vi "AlliGator Phasor Graph Actions.vi"(0 "AlliGator Q Elements in":T4[](array[typedef]), 1 "VI in":refnum<vi>, 2 "Script in":bool, 5 "Data Value Reference in":refnum<data-value>, 7 "AlliGator Q Event in":T5=enum."GUI:Idle", 9 "Data":variant, 11 "error in (no error)":errorcluster, 12 "AlliGator Ctrl Refnums":T6) -> (3 "Script out":bool, 4 "AlliGator Q Elements out":T4[](array[typedef]), 6 "Data Value Reference out":refnum<data-value>, 10 "[Notebook Message]":T1[](array[typedef]) {"Message Style"."Text Alignment" items=["Left", "Right", "Center"]}, 15 "error out":errorcluster)   [LabVIEW 2021, in "AlliGator Action Engine.lvlib"]
doc: "Processes AlliGator phasor graph-related actions."
uses:
  AlliGator Action Engine.lvlib
  AlliGator Internal Variables v2.ctl
  <vilib>/vision/Image Controls.llb/IMAQ Image.ctl
  AlliGator Gate Image Set.ctl
  AlliGator FLI Dataset Type.ctl
  AlliGator Data Series Type.ctl
  AlliGator Dataset Channel.ctl
  AlliGator Gate Arithmetic.ctl
  AlliGator Displayed Image.ctl
  Image/Named ROI Description.ctl
  AlliGator Decay Metadata v3.ctl
  AlliGator Decay Background Subtraction Info.ctl
  AlliGator Baseline Subtraction Method.ctl
  Graphs/XY Graph/XY Graph Plot Shift Parameters.ctl
  Graphs/XY Graph/XY Graph Plot Shift Method.ctl
  AlliGator Decay Extrapolation Parameters.ctl
  Phasor/Calibration Phasor (m, phi).ctl
  Phasor/Phasor Reference Series.ctl
  Phasor/Phasor Calibration Map v2.ctl
  Phasor/Phasor (g, s).ctl
  AlliGator Raw Phasor Plot Data v4.ctl
  Phasor/Phasor Standard Deviation Options.ctl
  AlliGator Phasor Multi-Harmonic Data.ctl
  Phasor/Phasor Harmonic Data.ctl
  AlliGator Decay Fit Options & Parameters v2.ctl
  Fits/IRF(X)PSED/Decay Fit Options v2.ctl
  Fits/Decay Convolution/Decay Model.ctl
  Fits/Residual Type.ctl
  Fits/IRF(X)PSED/Fit Weights Type.ctl
  Fits/Non-linear Fitting Method v2.ctl
  Fits/Fit Calculation Method.ctl
  Fits/Non-linear Fitting Algorithm.ctl
  AlliGator Decay Fit Parameter Constraints 2.ctl
  Fits/IRF(X)PSED/Decay Fit Parameters In List.ctl
  Fits/IRF(X)PSED/MLE Baseline Offset Type.ctl
  AlliGator Decay Preprocessing Parameters.ctl
  Fits/IRF(X)PSED/Decay Fit Parameters & Derived Quantities List.ctl
  AlliGator Q Event.ctl
  AlliGator Ctrl Refnums.ctl
  AlliGator Other Ctrl Refnums.ctl
  AlliGator State Indicator.ctl
  AlliGator Phasor Plot Ctrl Refnums.ctl
  AlliGator Phasor Graph Ctrl Refnums.ctl
  Phasor/Phasor Calibration Type.ctl
  AlliGator Dataset Ctrl Refnums.ctl
  AlliGator Registered Events Ctrl Refnums.ctl
  AlliGator Image Histogram Control Refnums.ctl
  Histograms/Linear Histogram Options.ctl
  Histograms/Histogram Bin Option.ctl
  Histograms/Histogram Bin Position.ctl
  AlliGator Decay Fit Map Control Refnums.ctl
  AlliGator Q Element.ctl
  Notebook/Notebook Message Object.ctl
  Rich Text Box/Text Formatting.ctl
  Rich Text Box/Text Colors.ctl
  Graphs/XY Graph/XY Graph Mouse Click Event Data.ctl
  Graphs/XY Graph/XY Graph Refnum.ctl
  <vilib>/Utility/miscctls.llb/LVPoint32TypeDef.ctl
  Graphs/XY Graph/XY Graph Selected Plot Info.ctl
  AlliGator Raw Phasor Plot Array Action.ctl
  Alligator Elements Order in Action Stack.ctl
  Graphs/XY Graph/New Plot Information.ctl
  Graphs/Plot Scales.ctl
  Graphs/LabVIEW Plot Interpolation.ctl
  Graphs/Plot Point Style.ctl
  AlliGator Variables List.ctl
  AlliGator Phasor Plot Scatter Plot Parameters.ctl
  AlliGator Phasor Graph Parameter List.ctl
  AlliGator Phasor Reference Data.ctl
  Phasor/Phasor (m, phi).ctl
  c0cd7910-0c77-40da-ae9a-85fce9394af2.vi
  da8c548c-3fe3-4ac5-84e2-54aef6c91d4f.vi
  Graphs/Get Plot at Mouse Click (XY Graph)/Get Plot at Mouse Click [AAC].vi
  AlliGator Add Single Action to Stack.vi
  AlliGator Add Action Array to Stack.vi
  Variant/Variant to Data/Variant to Boolean.vi
  Variant/Variant to Data/Variant to Path.vi
  Variant/Variant to Data/Variant to [Path].vi
  Arrays/Signed Array Index.vi
  Variant/Variant to Data/Variant to I32.vi
  <vilib>/Utility/error.llb/Error Cluster From Error Code.vi
  Variant/Variant to Data/Variant to U32.vi
  <userlib>/_OpenG.lib/array/array.llb/Filter 1D Array with Scalar (I32)__ogtk.vi
  <vilib>/ErrorRing/Error Ring.xnode
  GUI/GUI.lvlib
  AlliGator Scripts.lvlib
  Graphs/Graphs.lvlib
  Variant/Variant to Data/Variant to Data.lvlib
  AlliGator Phasor Graph.lvlib
  AlliGator Internal Variables.lvlib
  Graphs/XY Graph/XY Graph Add-Ons.lvlib
  Phasor/Phasor.lvlib
  AlliGator Phasor Ratio.lvlib
  Strings/Strings.lvlib
  <userlib>/_OpenG.lib/array/array.llb/openg_array.lvlib
  AlliGator Source Image.lvlib
  AlliGator Files.lvlib
  AlliGator Graphs.lvlib
  AlliGator Settings.lvlib
  Rich Text Box/Rich Text Box.lvlib
  Sound/Sound.lvlib
  Error/Error.lvlib
  AlliGator Globals, Variables & Constants.lvlib
  Image/Image.lvlib
  AlliGator Decay Preprocessing.lvlib
  AlliGator Phasor Plot.lvlib
  Fits/Fits.lvlib
  AlliGator Decay Fit.lvlib
  AlliGator Decay Fit Parameter Map.lvlib
  AlliGator GUI.lvlib
  AlliGator Dual-Channel Datasets.lvlib
  Histograms/Histogram Window.lvlib
  Notebook/Notebook.lvlib
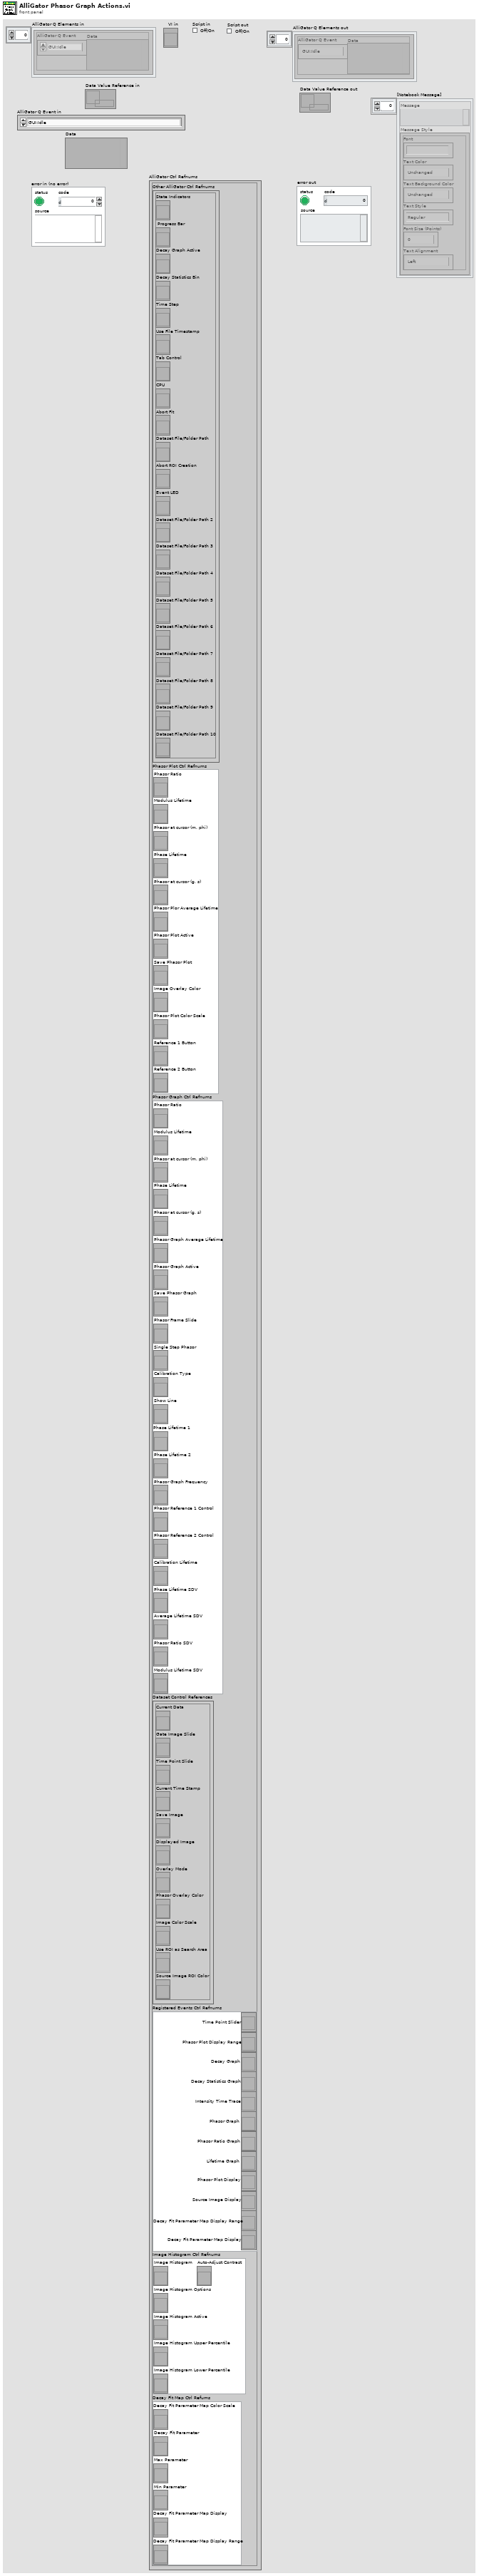
[diagram p1: front panel]
types:
  T1 = typedef "Notebook.lvlib/Notebook Message Object.ctl" = cluster{"Message":string, "Message Style":T2}
  T2 = typedef "Rich Text Box.lvlib/Text Formatting.ctl" = cluster{"Font":string, "Text Color":T3, "Text Background Color":T3, "Text Style":enum16{"Regular", "Bold", "Italic", "Underline", "Strikeout"}, "Font Size (Points)":dbl, "Text Alignment":i32}
  T3 = typedef "Rich Text Box.lvlib/Text Colors.ctl" = enum16{"Unchanged", "Black", "Blue", "Brown", "Gray", "Green", "Orange", "Pink", "Red", "White"}
  T4 = typedef "AlliGator Action Engine.lvlib/AlliGator Q Element.ctl" = cluster{"AlliGator Q Event":T5, "Data":variant}
  T5 = typedef "AlliGator Action Engine.lvlib/AlliGator Q Event.ctl" = enum16{"---- Files ----", "Files:Set Batch Export Files To Save", "Files:Set Dataset Loading & Pre-processing Options", "Files:Check #Frames in Dataset", "Files:Increment Frame Index", "Files:Open Mask Image", "Files:Open White Light Image", "Files:Open Single Dataset", "Files:New Folder of Folders Selected", "Files:Load File (all Types)_Scriptable", "Files:Move Flattened Series to Folders Series", "Files:Select Folder", "Files:Load FLI Dataset", "Files:Load Swiss SPAD 1 Dataset", "Files:Load Swiss SPAD 2 Dataset", "Files:Load .sdt FLI Dataset", "Files:Load .ptu FLI Dataset", "Files:Load .bin FLI Dataset", "Files:Load Single Gate Image Folder", "Files:Load I/m/phi Dataset (deprecated)", "Files:Load Single Image", "Files:Subtract Background File", "Files:Export FLI Dataset", "Files:Load HDF5 FLI Dataset", "Files:Set Destination File Path", "Files:Save Mask Image", "Files:Batch Conversion", "Files:New Folder Selected", "Files:Close FLI Dataset", "Files:Close FLI Dataset Series", "Files:Close White Light Image", "Files:Close Mask Image", "---- FLI Dataset ----", "FLI Dataset:Channel Arithmetic", "FLI Dataset:Export Average Lifetime Map as ASCII", "FLI Dataset:Export User-Defined Quantity Map as ASCII", "FLI Dataset:Python Function FLI Dataset Event", "FLI Dataset:ROI Analysis", "FLI Dataset:Tilted Logistic Square Gated IRF Characteristics Map", "FLI Dataset:Logistic Square Gated IRF Characteristics Map", "FLI Dataset:Square Gated IRF Characteristics Map", "FLI Dataset:Multi-ROI Single-Pixel Phasor Analysis", "FLI Dataset:Multi-ROI Single-Pixel NLSF Analysis", "FLI Dataset:All ROIs IRF Extraction", "FLI Dataset:All ROIs Decay Fit Non-Interactive (Fast + Individual IRF)", "FLI Dataset:All ROIs Phasor Analysis", "FLI Dataset:All ROIs Decay Fit", "FLI Dataset:Fluorescence Decay Statistics", "FLI Dataset:Update Decay Statistics Graph", "FLI Dataset:Get Decay from ROI", "FLI Dataset:All ROIs Average Lifetimes", "---- FLI Dataset Series ----", "FLI Dataset Series:Sum All Datasets in Series", "FLI Dataset Series:Add Dataset to Accumulated Dataset", "FLI Dataset Series:Display Accumulated Dataset", "FLI Dataset Series:Clear Dataset Series Sum", "FLI Dataset Series:Time-Series Analysis (NLSF)", "FLI Dataset Series:Time-Series Analysis (Phasor)", "---- Image ----", "Image:Update Image Profile Plots", "Image:Image Histogram Cursor Move", "Image:Image Histogram", "Image:Image Contrast", "Image:Set Image Histogram Cursor Move Flag", "Image:Clear Image Overlay", "Image:Use ROI as Search Area", "Image:Set ROI Diameter", "Image:Save Image Data as TIFF", "Image:Save Displayed Image with Overlay", "Image:Save Image Overlay Only", "Image:Save Image as Hot Pixel Mask", "Image:Change Source Image Color Palette", "Image:Copy Image to Clipboard", "Image:Source Image ROI Selection", "Image:Delete All ROIs", "Image:Delete All Unselected ROIs", "Image:Delete ROI", "Image:Merge All ROIs", "Image:Store ROI", "Image:Source Image ROI Storage", "Image:Export ROI Description to Notebook", "Image:Save ROI", "Image:Load ROI", "Image:Paste ROI Definition", "Image:Clear ROI", "Image:Identify ROIs in Mask Image", "Image:Create Complementary ROI", "Image:Create Contour ROI", "Image:Create ROI(s) from Pixels with Peak above Min_Scriptable", "Image:Create ROI(s) from Pixels with Intensity above Min_Scriptable", "Image:Compute ROI Statistics", "Image:Delete ROI(s) based on ROI Characteristics", "Image:Create ROI Grid", "Image:ROI to Individual Pixel ROIs", "Image:Python Function Source Image Event", "Image:Show Phasor Calibration Map ROI Centers", "Image:Convert ROI to Mask Image", "Image:Mouse Move", "Image:Mouse Up", "Image:Set Source Image Mouse Move Flag", "Image:Add Scale Bar Overlay", "Image:Delete Existing ROIs Option", "---- Decay ----", "Decay:Clear IRF/Reference Plot", "Decay:Clear Local IRFs", "Decay:Add Decay to Graph", "Decay:Smoothen Plot", "Decay:Smoothen Plot Tail", "Decay:Average Selected Plots", "Decay:Extract IRF", "Decay:Optimal IRF Extraction", "Decay:Threshold IRF", "Decay:Fit to Model IRF", "Decay:Fit IRF to Square Gate", "Decay:Fit IRF to Logistic Square Gate", "Decay:Fit IRF to Tilted Logistic Square Gate", "Decay:Create Bounding Cursors Set", "Decay:Export Bounding Cursors Definition to Notebook", "Decay:Denoise Plot", "Decay:Compute Cumulative Function", "Decay:Use as Reference Decay", "Decay:Show Reference Decay/IRF", "Decay:Extrapolate Decay", "Decay:Create Head & Tail Bounding Cursors", "Decay:Store Cursor-defined Head & Tail Fractions", "Decay:Rebin Plot", "Decay:1-Normalize Decay", "Decay:[0-1]-Normalize Plot", "Decay:Straighten Decay", "Decay:Shift Decay", "Decay:Fold Decay", "Decay:Fit Decay", "Decay:Global Fit of Selected Decays", "Decay:Post Global Fit Script", "Decay:Add Global Fit Parameters to Graph", "Decay:Add Decay Parameter(s) to Plot (Graph)", "Decay:Export Decay to Phasor Graph", "Decay:Plot Decay Shifts", "Decay:Compute Average Lifetime", "Decay:Plot Convolution", "Decay:Graph Tip Strip Update", "---- Decay Statistics ----", "Decay Statistics:Tip Strip Update", "---- Intensity Time Trace ----", "Intensity Time Trace:Use File Timestamp", "Intensity Time Trace:Load Intensity Corrections File", "Intensity Time Trace:Clear Intensity Corrections File", "Intensity Time Trace:Tip Strip Update", "---- Phasor Plot ----", "Phasor Plot:Build Phasor Plot", "Phasor Plot:Change Phasor Plot Color Palette", "Phasor Plot:Adjust Phasor Plot Display Range", "Phasor Plot:Highlight Image ROI in Phasor Plot", "Phasor Plot:Save Phasor Plot Image with Overlay", "Phasor Plot:Export Complex Phasor Map", "Phasor Plot:Export Phasor Ratio Map", "Phasor Plot:Export Average Lifetime Map", "Phasor Plot:Compute Phase Lifetime Histogram", "Phasor Plot:Compute Phasor Ratio Histogram", "Phasor Plot:Compute Phase Lifetime vs Intensity Scatter Plot", "Phasor Plot:Weber 2-Component Decomposition", "Phasor Plot:Update Phasor Color Map Vertices", "Phasor Plot:Clear Phasor Overlay", "Phasor Plot:Use Segment Extremities as References", "Phasor Plot:Use UC/Segment Intersections as References", "Phasor Plot:Use UC/Principal Axis Intersections as References", "Phasor Plot:Use UC/Linear Fit Intersections as References", "Phasor Plot:Update Phasor Plot Reference", "Phasor Plot:Show Local Phasor Info in Phasor Plot", "Phasor Plot:Update Phasor Plot State", "Phasor Plot:Phasor Plot ROI Storage", "Phasor Plot:Phasor Plot ROI Selection", "Phasor Plot:Python Function Phasor Plot Event", "Phasor Plot:Overlay Phasor ROI, Ratio or Map in Source Image", "Phasor Plot:Compute Decay of Selected Phasors", "Phasor Plot:Phasor at Image Pixel", "Phasor Plot:Mouse Move", "Phasor Plot:Mouse Up", "Phasor Plot:Display Range Mouse Move", "Phasor Plot:Set Mouse Move Flag", "---- Phasor Graph ----", "Phasor Graph:Calibrated Phasor Map Series", "Phasor Graph:Whole Image Phasor Scatter Plot (Todo)", "Phasor Graph:Get Phasor Value", "Phasor Graph:Create New Phasor Plot Dialog", "Phasor Graph:Update Last Phasor Value", "Phasor Graph:Update Phasor (m, phi)", "Phasor Graph:Remove Single Phasor from Plot", "Phasor Graph:Add Single Phasor to Plot", "Phasor Graph:Remove Phasor Plot", "Phasor Graph:Remove Selected Phasor Plots", "Phasor Graph:Clear Phasor Data", "Phasor Graph:Clear Phasor Graph", "Phasor Graph:Cursor Move", "Phasor Graph:Draw Cursor Connecting Line", "Phasor Graph:Clear Cursor Connecting Line", "Phasor Graph:Find UC Intersection", "Phasor Graph:Use UC/Cursor-Defined Line Intersections", "Phasor Graph:Use Selected Plots Fitted Line/UC Intersections", "Phasor Graph:Use Selected Plots Principal Axis/UC Intersections", "Phasor Graph:Show Single Phasor", "Phasor Graph:Save Single Phasor Plot", "Phasor Graph:Save All Phasor Plots", "Phasor Graph:Load Phasor Plot(s)", "Phasor Graph:Phasor Multiplication", "Phasor Graph:Compute Average Phasor", "Phasor Graph:Compute Multiple Average Phasors (Selected Plots)", "Phasor Graph:Export Single Phasor Plot Phase Lifetimes", "Phasor Graph:Phase Lifetime Trajectory", "Phasor Graph:Phase Lifetime vs Intensity Scatter Plot (deprecated)", "Phasor Graph:Parameter 2 vs Parameter 1 Scatter Plot", "Phasor Graph:Use Cursor n Location", "Phasor Graph:Set Reference n to Current Phase Lifetime Value", "Phasor Graph:Set Reference n to Lifetime Value", "Phasor Graph:Set Cursor n Location", "Phasor Graph:Save Phasor Graph Image", "Phasor Graph:Update SEPL Plot", "Phasor Graph:Export Single Phasor Plot Data", "Phasor Graph:Export Selected Phasor Plots Data", "Phasor Graph:Python Function Phasor Graph Event", "Phasor Graph:Tip Strip Update", "---- Calibration ----", "Calibration:Set Calibration Type", "Calibration:Load/Save Phasor Calibration", "Calibration:Load/Save Phasor Calibration Series", "Calibration:Load/Save Phasor Calibration Map", "Calibration:Use as Calibration", "Calibration:Compute Optimal Calibration from Phasor References", "Calibration:Clear Phasor Calibration", "Calibration:Single Phasor Calibration Information", "Calibration:Use as Calibration Series", "Calibration:Use as Calibration Map", "Calibration:Clear Calibration Series", "Calibration:Phasor Calibration Series Information", "Calibration:Clear Calibration Map", "Calibration:Phasor Calibration Map Information", "Calibration:Apply Phasor Calibration", "Calibration:Update Single Plot Calibration", "Calibration:Update Multiple Plots Calibration", "Calibration:Clear Single Plot Calibration", "Calibration:Clear All Plots Calibrations", "Calibration:Clear Plot(s) Calibration(s)?", "Calibration:Phasor Calibration Maps (# Gates Series)", "---- Phasor Ratio ----", "Phasor Ratio:Clear Reference n", "Phasor Ratio:Toggle Selected Plot(s)  Lock to Reference 1", "Phasor Ratio:Use as Reference n", "Phasor Ratio:Send Reference n to Notebook", "Phasor Ratio:Toggle Selected Plot(s)  Lock to Reference 2", "Phasor Ratio:Compute Phasor Ratio at Mouse Location", "Phasor Ratio:Compute Phasor Plot's Average Phasor Ratio", "Phasor Ratio:Compute Time-Series Phasor Ratios", "Phasor Ratio:Fit Line to Phasor Ratio Plot", "Phasor Ratio:Save References", "Phasor Ratio:Load References", "Phasor Ratio:Update Phasor Reference 1", "Phasor Ratio:Update Phasor Reference 2", "Phasor Ratio:Move Cursor n to Reference n", "Phasor Ratio:Use as Phasor Reference 1 Lifetime", "Phasor Ratio:Use as Phasor Reference 2 Lifetime", "Phasor Ratio:Export Phasor Ratio Map as ASCII", "Phasor Ratio:Tip Strip Update", "---- Lifetime & Other Parameters Graph ----", "Lifetime:Tip Strip Update", "---- Decay Fit Parameter Map ----", "Decay Fit Parameter Map:Export ROI NLSF Data as ASCII", "Decay Fit Parameter Map:Set Decay Fit  Parameter Map Selection", "Decay Fit Parameter Map:Build Decay Fit Parameter Map", "Decay Fit Parameter Map:Change Decay Fit Parameter Map Color Palette", "Decay Fit Parameter Map:Export Decay Fit Parameter Map Data as ASCII", "Decay Fit Parameter Map:Export All Decay Fit Parameter Maps Data as ASCII", "Decay Fit Parameter Map:Send Map Data to Lifetime Graph", "Decay Fit Parameter Map:Save Decay Fit Parameter Map Image", "Decay Fit Parameter Map:Save-Load IRFs & Fit Data", "Decay Fit Parameter Map:Update Local Decay Plots", "Decay Fit Parameter Map:Python Function Decay Fit Parameters Map Event", "Decay Fit Parameter Map:Overlay Decay Fit Parameter Map in Source Image", "Decay Fit Parameter Map:Plot Map Data vs Intensity", "Decay Fit Parameter Map:Mouse Up", "Decay Fit Parameter Map:Display Range Mouse Move", "---- Generic Graph ----", "Generic Graph:Generic XY Graph Event", "Generic Graph:Python Function XY Graph Event", "Generic Graph:New Plot", "Generic Graph:Save Plot", "Generic Graph:XY Plot Histogram", "Generic Graph:Set XY Graph Plot Name", "Generic Graph:Set Last Cursor Style", "Generic Graph:Tip Strip Update", "---- GUI ----", "GUI:Start Script", "GUI:Type of Displayed Image Changed", "GUI:Gate Image Slide Changed", "GUI:Show Busy Icon", "GUI:Show Busy Icon & Abort Button", "GUI:Hide Busy Icon", "GUI:Hide Busy Icon & Abort Button", "GUI:Abort", "GUI:End Script", "GUI:Start Timing", "GUI:End Timing", "GUI:Set State Indicator", "GUI:Send Parameters JSON Strings to Clipboard", "GUI:Set Gate Step", "GUI:Idle", "GUI:Initialization", "GUI:Quit", "GUI:Increment Dataset Index", "GUI:Set Dataset Index to -1", "GUI:Time Series Slider Moved", "GUI:Time Series Slider Changed", "GUI:Toggle Playback or Loop", "GUI:Playback Script", "GUI:Set Phasor Frequency", "GUI:Open Window", "GUI:Start Test Script", "GUI:End Test Script", "DEBUG"}
  T6 = typedef "AlliGator GUI.lvlib/AlliGator Ctrl Refnums.ctl" = cluster{"Other AlliGator Ctrl Refnums":T7, "Phasor Plot Ctrl Refnums":T8, "Phasor Graph Ctrl Refnums":T9, "Dataset Control References":T10, "Registered Events Ctrl Refnums":T11, "Image Histogram Ctrl Refnums":T12, "Decay Fit Map Ctrl Refums":T13}
  T7 = typedef "AlliGator GUI.lvlib/AlliGator Other Ctrl Refnums.ctl" = cluster{"State Indicators":refnum<vi>, " Progress Bar":refnum<vi>, "Decay Graph Active":refnum<vi>, "Decay Statistics Bin":refnum<vi>, "Time Step":refnum<vi>, "Use File Timestamp":refnum<vi>, "Tab Control":refnum<vi>, "CPU":refnum<vi>, "Abort Fit":refnum<vi>, "Dataset File/Folder Path":refnum<vi>, "Abort ROI Creation":refnum<vi>, "Event LED":refnum<vi>, "Dataset File/Folder Path 2":refnum<vi>, "Dataset File/Folder Path 3":refnum<vi>, "Dataset File/Folder Path 4":refnum<vi>, "Dataset File/Folder Path 5":refnum<vi>, "Dataset File/Folder Path 6":refnum<vi>, "Dataset File/Folder Path 7":refnum<vi>, "Dataset File/Folder Path 8":refnum<vi>, "Dataset File/Folder Path 9":refnum<vi>, "Dataset File/Folder Path 10":refnum<vi>}
  T8 = typedef "AlliGator GUI.lvlib/AlliGator Phasor Plot Ctrl Refnums.ctl" = cluster{"Phasor Ratio":refnum<vi>, "Modulus Lifetime":refnum<vi>, "Phasor at cursor (m, phi)":refnum<vi>, "Phase Lifetime":refnum<vi>, "Phasor at cursor (g, s)":refnum<vi>, "Phasor Plor Average Lifetime":refnum<vi>, "Phasor Plot Active":refnum<vi>, "Save Phasor Plot":refnum<vi>, "Image Overlay Color":refnum<vi>, "Phasor Plot Color Scale":refnum<vi>, "Reference 1 Button":refnum<vi>, "Reference 2 Button":refnum<vi>}
  T9 = typedef "AlliGator GUI.lvlib/AlliGator Phasor Graph Ctrl Refnums.ctl" = cluster{"Phasor Ratio":refnum<vi>, "Modulus Lifetime":refnum<vi>, "Phasor at cursor (m, phi)":refnum<vi>, "Phase Lifetime":refnum<vi>, "Phasor at cursor (g, s)":refnum<vi>, "Phasor Graph Average Lifetime":refnum<vi>, "Phasor Graph Active":refnum<vi>, "Save Phasor Graph":refnum<vi>, "Phasor Frame Slide":refnum<vi>, "Single Step Phasor":refnum<vi>, "Calibration Type":refnum<vi>, "Show Line":refnum<vi>, "Phase Lifetime 1":refnum<vi>, "Phase Lifetime 2":refnum<vi>, "Phasor Graph Frequency":refnum<vi>, "Phasor Reference 1 Control":refnum<vi>, "Phasor Reference 2 Control":refnum<vi>, "Calibration Lifetime":refnum<vi>, "Phase Lifetime SDV":refnum<vi>, "Average Lifetime SDV":refnum<vi>, "Phasor Ratio SDV":refnum<vi>, "Modulus Lifetime SDV":refnum<vi>}
  T10 = typedef "AlliGator GUI.lvlib/AlliGator Dataset Ctrl Refnums.ctl" = cluster{"Current Data":refnum<vi>, "Gate Image Slide":refnum<vi>, "Time Point Slide":refnum<vi>, "Current Time Stamp":refnum<vi>, "Save Image":refnum<vi>, "Displayed Image":refnum<vi>, "Overlay Mode":refnum<vi>, "Phasor Overlay Color":refnum<vi>, "Image Color Scale":refnum<vi>, "Use ROI as Search Area":refnum<vi>, "Source Image ROI Color":refnum<vi>}
  T11 = typedef "AlliGator GUI.lvlib/AlliGator Registered Events Ctrl Refnums.ctl" = cluster{"Time Point Slider":refnum<vi>, "Phasor Plot Display Range":refnum<vi>, "Decay Graph":refnum<vi>, "Decay Statistics Graph":refnum<vi>, "Intensity Time Trace":refnum<vi>, "Phasor Graph":refnum<vi>, "Phasor Ratio Graph":refnum<vi>, "Lifetime Graph":refnum<vi>, "Phasor Plot Display":refnum<vi>, "Source Image Display":refnum<vi>, "Decay Fit Parameter Map Display Range":refnum<vi>, "Decay Fit Parameter Map Display":refnum<vi>}
  T12 = typedef "AlliGator GUI.lvlib/AlliGator Image Histogram Control Refnums.ctl" = cluster{"Image Histogram":refnum<vi>, "Image Histogram Options":refnum<vi>, "Image Histogram Active":refnum<vi>, "Image Histogram Upper Percentile":refnum<vi>, "Image Histogram Lower Percentile":refnum<vi>, "Auto-Adjust Contrast":refnum<vi>}
  T13 = typedef "AlliGator Decay Fit Parameter Map.lvlib/AlliGator Decay Fit Map Control Refnums.ctl" = cluster{"Decay Fit Parameter Map Color Scale":refnum<vi>, "Decay Fit Parameter":refnum<vi>, "Max Parameter":refnum<vi>, "Min Parameter":refnum<vi>, "Decay Fit Parameter Map Display":refnum<vi>, "Decay Fit Parameter Map Display Range":refnum<vi>}
  T14 = typedef "XY Graph Add-Ons.lvlib/XY Graph Selected Plot Info.ctl" = cluster{"Multiplot XY Graph":T15, "Mouse Coordinates":T16, "Plot Index":i32}
  T15 = typedef "XY Graph Add-Ons.lvlib/XY Graph Refnum.ctl" = refnum<vi>
  T16 = typedef "LVPoint32TypeDef.ctl" = cluster{"Horizontal":i32, "Vertical":i32}
  T17 = typedef "XY Graph Add-Ons.lvlib/XY Graph Mouse Click Event Data.ctl" = cluster{"Multiplot XY Graph":T15, "Mouse Coordinates":T16}
  T18 = typedef "Phasor.lvlib/Calibration Phasor (m, phi).ctl" = cluster{"m":dbl, "phi":dbl, "Phasor Frequency":dbl[unit], "Reference Lifetime":dbl[unit]}
  T19 = typedef "AlliGator Phasor Graph.lvlib/AlliGator Raw Phasor Plot Array Action.ctl" = enum16{"Clear All", "-", "Add Raw Phasor Plot", "Delete Raw Phasor Plot", "Replace Raw Phasor Plot", "---------------------", "Add Phasor to Plot", "Replace Phasor in Plot", "Remove Phasor in Plot"}
  T20 = typedef "AlliGator Action Engine.lvlib/Alligator Elements Order in Action Stack.ctl" = enum16{"Enqueue 2 AFTER 1", "Enqueue 2 BEFORE 1"}
  T21 = typedef "XY Graph Add-Ons.lvlib/New Plot Information.ctl" = cluster{"Multiplot XY Graph":refnum<vi>, "Plot Name":string, "Plot Scales":T22, "Plot Interpolation":T23, "Point Style":T24, "Plot Color":u32, "Plot Metadata":variant}
  T22 = typedef "XY Graph Add-Ons.lvlib/Plot Scales.ctl" = cluster{"X Scale":u32, "Y Scale":u32}
  T23 = typedef "Graphs.lvlib/LabVIEW Plot Interpolation.ctl" = u8
  T24 = typedef "Graphs.lvlib/Plot Point Style.ctl" = enum16{"not defined", "None", "Empty Circle", "Filled Circle", "Thick Circle", "Dotted Circle", "Empty Square", "Filled Square", "Thick Square", "Dotted Square", "Small Filled Square", "Dot", "Cross", "Tiny Cross", "Large X", "Small x", "Diamond", "Small Empty Square"}
  T25 = typedef "AlliGator Globals, Variables & Constants.lvlib/AlliGator Variables List.ctl" = enum16{"---- GUI ----", "Initialization Status", "State Indicators Refnum", "Original AlliGator Menu Items", "Current Action Loop State", "Script in progress", "Playback", "Loop Playback", "Search ROI Used", "Search ROI", "Decay Graph Max Legend Size", "Intensity Graph Max Legend Size", "Decay Statistics Graph Max Legend Size", "Phasor Graph Max Legend Size", "Phasor Ratio Graph Max Legend Size", "Lifetime Graph Max Legend Size", "---- Files ----", "Export Dataset Frames as Individual Files", "Show Batch Export Help Balloons", "Frames in Dataset", "ptu File Frame Start Indices", "Current Frame in Dataset", "Current Frame Timestamp", "------ Python Plugins ------", "Python Plugins Information", "Python Session", "Valid Python Session?", "---- Source Image ----", "Dataset Loaded", "Dataset Metadata", "Dataset Channel", "Dataset Data Description", "Background Dataset Metadata", "Background Dataset Channel", "Background Dataset Data Description", "Background File Subtraction", "Background File Path", "Background File Pile-up Correction", "Background File Pixel Well Capacity", "Background File Scaling Factor", "Source Image ROIs", "Current Source Image ROI", "Source Image ROI Event Refnum", "X_Source Image Display Range", "X_Source Image Palette Information", "Source Image Palette List", "Source Image Scale", "Current Dataset Load Settings", "Source Image:ROI Overlay Color", "---- Image Profile Window ----", "Image Profile:Overlay ROI in Source Image", "Image Profile Window Event Refnum", "Image Profile:IntensityType", "Image Profile:Intensity Average Type", "Image Profile:Intensity-weighted SDV", "Image Profile:Box Profile Type", "Image Profile Window Open", "Image Profile:Plotted Fit Parameter", "X_Type of Displayed Image", "X_Time Gate Slider", "Dataset Path", "Source Image Overlay to Erase", "Is Displayed Image Accumulated", "White Light Image Modified", "Mask Image Modified", "Macrotime Gate Separation", "------ Phasor Graph -------", "Phasor Graph:Show Line", "---- Phasor Plot ---", "Phasor Plot Parameters Changed", "FLI Dataset Modified since last Phasor Plot Calculation", "Phasor Harmonics Data", "Selected Phasor Harmonics", "Phasor Harmonic Manager Event Refnum", "Phasor Plot ROIs", "Current Phasor Plot ROI", "Phasor Plot ROI Event Refnum", "Phasor Plot Image Reference Points", "Phasor Plot Computed", "Phasor Plot Palette Information", "Phasor Plot Palette List", "Phasor Ratio Palette Information", "Phasor Ratio Palette List", "Phasor Image Scale", "Phasor Plot Image Overlay to Erase", "Phasor Plot Image Elements to Update", "Current Phasor Plot Calculation Parameters", "Current Phasor Calibration Options", "Reset Cumulated Phasor Plot", "Phasor Ratio Reference 1", "Phasor Ratio Lifetime Reference 1", "Phasor Ratio Reference 1 Frequency", "Phasor Ratio Reference 2", "Phasor Ratio Lifetime Reference 2", "Phasor Ratio Reference 2 Frequency", "---- Decay Analysis ----", "Number of Selected Decays to Fit", "LS Fit Results", "LAR Fit Results", "BS Fit Results", "Last Decay Max - Min", "Best Fit Parameters", "Best Fit Parameter Names", "Actual Size X", "Actual Size Y", "Binning X", "Binning Y", "Actual # Gates", "Dataset Number", "Gates to...", "Gates Skipped", "Gates to keep", "Gate Step", "Gate Separation", "Reversed Gates", "Pile-up Correction", "Pixel Well Capacity", "Background Subtracted", "Background Subtraction Method", "Background Definition Range", "Background File (deprecated)", "Number of Dataset Accumulated", "Array of Accumulated Dataset Paths", "Do Averaged Datasets", "Destination File Path", "Process Plot Target", "Use 1/D as Phasor Frequency", "---- Decay Fit Parameter Map -----", "Decay Fit Parameter Map Palette Information", "Decay Fit Parameter Map Palette List", "Local Decay Graph Window Event Refnum", "------- Local Decay Window ---------", "Use normalized IRF for convolution", "----- Miscellaneous ----", "Skippable Dialog Windows Status"}
  T26 = cluster{"Mouse Click Event Data":T17, "Save as...":bool}
  T27 = typedef "AlliGator Phasor Graph.lvlib/AlliGator Phasor Plot Scatter Plot Parameters.ctl" = cluster{"Parameter 2":T28, "Parameter 1":T28}
  T28 = typedef "AlliGator Phasor Graph.lvlib/AlliGator Phasor Graph Parameter List.ctl" = enum16{"Time Stamp", "Index", "Phasor Parameters", "Phasor g", "Phasor s", "Phasor phi", "Phasor m", "Modulus Lifetime", "Phase Lifetime", "ROI Parameters", "ROI Center x", "ROI Center y", "ROI # pixels ", "Decay Parameters", "Intensity", "Background/Gate", "Intensity - Background", "Fitted Lifetime", "Fitted Intensity", "Phasor Ratio Parameters", "Amplitude Phasor Ratio", "Intensity Phasor Ratio", "Amplitude-Averaged Lifetime", "Intensity-Averaged Lifetime", "-", "Phasor Parameters SDV", "Phasor g SDV", "Phasor s SDV", "Phasor phi SDV", "Phasor m SDV", "Phase Lifetime SDV", "Modulus Lifetime SDV", "Phasor Ratio Parameters SDV", "Amplitude Phasor Ratio SDV", "Intensity Phasor Ratio SDV", "Amplitude-Averaged Lifetime SDV", "Intensity-Averaged Lifetime SDV"}
  T29 = typedef "Phasor.lvlib/Phasor (g, s).ctl" = cluster{"g":dbl, "s":dbl}
  T30 = cluster{"Current Phasor (g, s)":T29, "Cursor Id":u32}
  T31 = typedef "AlliGator Phasor Ratio.lvlib/AlliGator Phasor Reference Data.ctl" = cluster{"Data Type":string, "Data":variant}
  T32 = typedef "Phasor.lvlib/Phasor (m, phi).ctl" = cluster{"m":dbl, "phi":dbl}
  T33 = typedef "AlliGator Internal Variables.lvlib/AlliGator Internal Variables v2.ctl" = cluster{"Displayed Image":T34, "White Light Image":T34, "Mask Image":T34, "ROI Mask Image":T34, "Current Dataset Images 1":T35, "Background Dataset Images 1":T35, "Current Dataset Images 2":T35, "Background Dataset Images 2":T35, "Current Dataset Arithmetic Images":T35, "Accumulated Dataset Images 1":T35, "Accumulated Dataset Images 2":T35, "Accumulated Dataset Arithmetic Images":T35, "Phasor Plot Image":T34, "Decay Fit Parameter Map Image":T34, "Single Data Point Path":path, "White Light Image Path":path, "Mask Image Path":path, "Time-Series Folder":path, "[Time-Series Paths]":path[], "Current Dataset":i32, "Single Dataset Type":T36, "Current Folder":string, "AlliGator Data Series Type":T37, "# Datasets":i32, "Dual-Channel Dataset":bool, "Selected Channel Name":string, "Dataset Channel":T38, "Channel Arithmetic":T39, "Dual-Channel Background Dataset":bool, "Background Channel":T38, "Dual-Channel Accumulated Dataset":bool, "Start Time":dbl, "[Time-Series Timestamps]":dbl[], "[Intensity Corrections]":dbl[], "Time Series Script":bool, "Type of Displayed Image":T40, "Gate Image Slide":u16, "# Gates":i32, "ROIs":T41[], "ROI Decay":cluster{"t Array":dbl[], "I Array":dbl[]}, "Valid Decay":bool, "Decay  Metadata":T43, "Reference Decay Plot Name":string, "Reference Decay":cluster{"t Array":dbl[], "I Array":dbl[]}, "Decay Shift Plot":cluster{"Time Stamps":dbl[], "Decay Shifts":dbl[]}, "[Decays Max Values]":sgl[], "[Decays Min Values]":sgl[], "Calibration Phasor":T18, "Calibration Phasor Series":T49, "Phasor Calibration Map":T50, "Calibration Map MD5 Digest":string, "Last Raw Phasor":T29, "Last Calibrated Phasor":T29, "Last Calibrated Phasor SDV":T29, "Phasor Graph:Phasor Plot":cluster{"g Array":dbl[], "s Array":dbl[]}, "Phasor Graph:Phasor SDV Plot":cluster{"g Array":dbl[], "s Array":dbl[]}, "[Phasor Graph:Raw Phasor Plots]":T51[], "Phasor Plot locked to Ref 1":i32, "[Phasor Plot(s) locked to Ref 1]":i32[], "[Phasor Plot(s) locked to Ref 2]":i32[], "[Pixel Phasors]":T29[], "[[Sum Image]]":dbl[][], "[[CSG Phasors]]":csg[][], "[[Valid Pixel?]]":bool[][], "I/m/phi Dataset":cluster{"I/m/phi Dataset?":bool, "Base Frequency":dbl[unit], "Harmonic Orders":u8[]}, "Multi Phasor Plot Data":T53, "Decay Fit Options & Parameters":T55, "Fit Options: Decay Preprocessing Parameters":T66, "Fit Options: Reference Decay":cluster{"t Array":dbl[], "I Array":dbl[]}, "Is Full Image Parameters Map":bool, "Is Single-Pixels Parameters Map":bool, "NLSF Parameters Map X Resolution":i32, "NLSF Parameters Map Y Resolution":i32, "[Single Decay Fit Parameters]":dbl[], "Fit Model":T57, "[[Multiple Decays Fit Parameters]]":dbl[][], "[[Multiple Decays Fit Parameter SDVs]]":dbl[][], "[[IRFs]]":dbl[][], "IRF Array Time Axis":dbl[], "Decay Array Time Axis":dbl[], "[Decay Fit Parameter Names]":T67[], "[[Phasor Ratios]]":dbl[][], "[[Average Lifetimes]]":dbl[][], "Amplitude Weighted Average Lifetime":bool, "[Decay Sum]":dbl[], "[[User-defined Quantities]]":dbl[][], "User-defined Quantity":string}
  T34 = typedef "IMAQ Image.ctl" = refnum<image>
  T35 = typedef "AlliGator Internal Variables.lvlib/AlliGator Gate Image Set.ctl" = cluster{"SGL Image Max":T34, "SGL Image Sum":T34, "SGL Gate Images":T34[], "SGL Image Min":T34}
  T36 = typedef "AlliGator Files.lvlib/AlliGator FLI Dataset Type.ctl" = enum16{"HDF5 FLI Dataset", "Gate Image Folder", ".sdt FLI Dataset (Becker & Hickl)", ".ptu FLI Dataset (PicoQuant)", "SS1 FLI Dataset", "SS2 FLI Dataset", "I/m/phi Dataset", ".bin FLI Dataset (PicoQuant Binned)", ".bin FLI Dataset (Piccolo Binned)"}
  T37 = typedef "AlliGator Files.lvlib/AlliGator Data Series Type.ctl" = enum16{"Not a Supported Series", "Gate Images Folder Series", "SwissSPAD 2 Dataset Series", "B&H FLI Dataset Series", "PicoQuant PTU FLI Dataset Series", "PicoQuant BIN FLI Dataset Series", "Piccolo hist BIN FLI Dataset Series", "HDF5 FLI Dataset Series"}
  T38 = typedef "AlliGator Dual-Channel Datasets.lvlib/AlliGator Dataset Channel.ctl" = enum16{"G2", "INT"}
  T39 = typedef "AlliGator Settings.lvlib/AlliGator Gate Arithmetic.ctl" = enum16{"None", "INT-G2", "G2/INT*<INT>", "(1 - G2/INT)*<INT>"}
  T40 = typedef "AlliGator Source Image.lvlib/AlliGator Displayed Image.ctl" = enum16{"Single Gate", "Sum of All Gates", "Max of All Gates", "Min of All Gates", "-", "White Ligth Image", "Mask Image"}
  T41 = typedef "Image.lvlib/Named ROI Description.ctl" = cluster{"ROI Descriptor":T42, "ROI Name":string, "Overlay Color":u32}
  T42 = typedef "ROI Descriptor" = cluster{"Global Rectangle":i32[], "Contours":cluster{"ID":enum32{"External", "Internal"}, "Type":u32, "Coordinates":i32[]}[]}
  T43 = typedef "AlliGator Phasor Graph.lvlib/AlliGator Decay Metadata v3.ctl" = cluster{"ROI Descriptor":T42, "ROI Center":cluster{"X":i32, "Y":i32}, "Decay Background Subtraction Info":T44, "Decay Reverted":bool, "Decay Smoothened":bool, "Decay Straightened":bool, "Fitted Tau (Decay Straightening)":dbl, "Decay Shift Parameters":T46, "Decay Shifted":bool, "Decay Extrapolated":bool, "Decay Extrapolation Parameters":T48, "Decay Normalized":bool, "Fold Decay":bool, "# Folds":u32}
  T44 = typedef "AlliGator Decay Analysis.lvlib/AlliGator Decay Preprocessing.lvlib/AlliGator Decay Background Subtraction Info.ctl" = cluster{"Laser Period":dbl[unit], "Gate Duration":dbl[unit], "Baseline Subtraction Method":T45, "Background Definition Range":cluster{"Min Gate":dbl[unit], "Max Gate":dbl[unit]}, "Total Intensity w/o Bkgd Subtraction":dbl, "Bkgd-subtracted Intensity (exp)":dbl, "# Data Points":i32, "Background/Gate":dbl, "Fitted Lifetime":dbl[unit], "Bkgd-subtracted Intensity (theo)":dbl}
  T45 = typedef "AlliGator Decay Analysis.lvlib/AlliGator Decay Preprocessing.lvlib/AlliGator Baseline Subtraction Method.ctl" = enum16{"Mean", "Min", "Square Gated Single-Exponential", "File", "Constant"}
  T46 = typedef "XY Graph Add-Ons.lvlib/XY Graph Plot Shift Parameters.ctl" = cluster{"Type":T47, "Shift":dbl[unit], "Threshold":dbl, "Rotate":bool}
  T47 = typedef "XY Graph Add-Ons.lvlib/XY Graph Plot Shift Method.ctl" = enum16{"Default", "CFD", "Threshold", "Cross-Correlation"}
  T48 = typedef "AlliGator Decay Analysis.lvlib/AlliGator Decay Preprocessing.lvlib/AlliGator Decay Extrapolation Parameters.ctl" = cluster{"Additional Points":u32, "Head Fraction":dbl, "Fitted Tau":dbl, "Use Periodicity":bool, "Use Cursors":bool, "Tail Fraction":dbl}
  T49 = typedef "Phasor.lvlib/Phasor Reference Series.ctl" = cluster{"m Array":dbl[], "phi Array":dbl[], "Phasor Frequency":dbl[unit], "Calibration Lifetime":dbl[unit]}
  T50 = typedef "Phasor.lvlib/Phasor Calibration Map v2.ctl" = cluster{"Phasor Frequency":dbl[unit], "Calibration Lifetime":dbl[unit], "ROI Centers":cluster{"X":i32, "Y":i32}[], "ROI Descriptors":T42[], "Map Resolution X":i32, "Map Resolution Y":i32, "z Array":cdb[]}
  T51 = typedef "AlliGator Phasor Graph.lvlib/AlliGator Raw Phasor Plot Data v4.ctl" = cluster{"Phasor Plot Name":string, "Raw Phasor Plot":T29[], "Phasor Frequency":dbl[unit], "[Decay Metadata]":T43[], "Raw Phasor Plot SDV":T29[], "Phasor SDV Options":T52, "[Calibration Phasor]":T18[]}
  T52 = typedef "Phasor.lvlib/Phasor Standard Deviation Options.ctl" = cluster{"Compute Estimated SDV":bool, "# Replicas":u32, "Use Estimated Average Phasor":bool}
  T53 = typedef "AlliGator Phasor Plot.lvlib/AlliGator Phasor Multi-Harmonic Data.ctl" = cluster{"Base Frequency":dbl[unit], "# Harmonics":u8, "Harmonic Orders":u8[], "Phasor Plot Settings Checksum":u64, "Phasor Harmonic Data Array":T54[]}
  T54 = typedef "Phasor.lvlib/Phasor Harmonic Data.ctl" = cluster{"Phasor Harmonic Name":string, "Phasor Plot Settings Checksum":u64, "Phasor Frequency":dbl[unit], "Base Frequency":dbl[unit], "Harmonic Order":u8, "Phasor Plot Parameters":string, "Phasor Array [[CSG]]":csg[][], "Dataset File Path":path}
  T55 = typedef "AlliGator Decay Fit Parameter Map.lvlib/AlliGator Decay Fit Options & Parameters v2.ctl" = cluster{"SYNC Period":dbl[unit], "Fit Options":T56, "Fit Parameter Constraints":T63[], "MLE Baseline Offset":dbl, "MLE Baseline Offset Type":T65}
  T56 = typedef "Fits.lvlib/Decay Fit Options v2.ctl" = cluster{"Show Fit Residuals":bool, "Fit Model":T57, "Residual Type":T58, "Max Decay Percentile":dbl, "Min Decay Percentile":dbl, "Show Full Decay":bool, "Weights":T59, "Fitting Method":T60, "Compute Parameter Uncertainties":bool, "Periodic Boundaries":bool, "Model Calculation":T61, "Period":dbl[unit], "Termination Criteria":cluster{"Max Iterations":i32, "Max Function Calls":i32, "Max Time":dbl[unit], "Function Tolerance":dbl, "Parameter Tolerance":dbl, "Gradient Tolerance":dbl, "Min Lambda":dbl, "Max Lambda":dbl, "Initial Tick Count":u32}, "Offset Resolution":dbl[unit], "Use Local IRF":bool, "Fitting Algorithm":T62}
  T57 = typedef "Fits.lvlib/Decay Model.ctl" = enum16{"1-Exponential", "2-Exponentials"}
  T58 = typedef "Fits.lvlib/Residual Type.ctl" = enum16{"Standard", "Normalized", "Reduced"}
  T59 = typedef "Fits.lvlib/Fit Weights Type.ctl" = enum16{"Unweighted", "1/Variance", "Best of All"}
  T60 = typedef "Fits.lvlib/Non-linear Fitting Method v2.ctl" = enum16{"Least Square", "Least Absolute Residual", "Bisquare", "MLE", "-", "Best of All"}
  T61 = typedef "Fits.lvlib/Fit Calculation Method.ctl" = enum16{"Simulation", "Convolution", "Integration"}
  T62 = typedef "Fits.lvlib/Non-linear Fitting Algorithm.ctl" = enum16{"Levenberg-Marquardt", "Trust-Region Dogleg"}
  T63 = typedef "AlliGator Decay Analysis.lvlib/AlliGator Decay Fit.lvlib/AlliGator Decay Fit Parameter Constraints 2.ctl" = cluster{"Fit Parameter":T64, "Min Value":dbl, "Max Value":dbl, "Global":bool, "Used":bool}
  T64 = typedef "Fits.lvlib/Decay Fit Parameters In List.ctl" = enum16{"Offset", "Baseline", "A_1", "tau_1", "A_2", "tau_2"}
  T65 = typedef "Fits.lvlib/MLE Baseline Offset Type.ctl" = enum32{"Absolute", "Percentage"}
  T66 = typedef "AlliGator Decay Analysis.lvlib/AlliGator Decay Preprocessing.lvlib/AlliGator Decay Preprocessing Parameters.ctl" = cluster{"Background Subtraction":bool, "Straighten Decay":bool, "Reverse Gates":bool, "1-Normalized Decay":bool, "Smoothen Decay":bool, "Smoothing Parameter":dbl, "Shift Decay":bool, "Decay Shift Parameters":T46, "Extrapolate Decay":bool, "Additional Points":u32, "Head Fraction":dbl, "Pixel-Normalize Decay":bool, "Use Periodicity":bool, "Use Cursors":bool, "Tail Fraction":dbl, "Use Decay Pre-Processing":bool, "Fold Decay":bool, "# Folds":u32, "[0-1]-Normalized Decay":bool}
  T67 = typedef "Fits.lvlib/Decay Fit Parameters & Derived Quantities List.ctl" = enum16{"Offset", "Baseline", "A_1", "tau_1", "A_2", "tau_2", "<tau>_a", "f1_a", "f2_a", "<tau>_i", "f1_i", "f2_i", "-", "R^2", "Chi^2"}
  T68 = typedef "AlliGator Scripts.lvlib/AlliGator Dataset + Calibration Map + Gate Step.ctl" = cluster{"Phasor Calibration Map Path":path, "Gate Step":i32, "Dataset Path":path}
  T69 = cluster{"Selected Plot Info":T14, "Scatter Plot Parameters":T27}
  T70 = typedef "AlliGator Phasor Graph.lvlib/AlliGator Phasor Plot Destination.ctl" = enum32{"Phasor Plot 1", "Phasor Plot 2", "New Phasor Plot"}
  T71 = typedef "AlliGator Phasor Graph.lvlib/AlliGator 2-Phasor Plot Multiplication.ctl" = cluster{"Phasor Plot 1":u16, "Operation 1":T72, "Phasor Plot 2":u16, "Operation 2":T72, "Delay":dbl[unit], "Operation 3":T72, "1-Exp Lifetime":dbl[unit], "Operation 4":T72, "Phasor (g, s)":T29, "Phasor (m, phi)":T32, "Phasor Representation":T73, "Use Operation 1":bool, "Use Operation 2":bool, "Use Operation 3":bool, "Use Operation 4":bool}
  T72 = typedef "Phasor.lvlib/Phasor Operation.ctl" = enum16{"*", "/"}
  T73 = typedef "Phasor.lvlib/Phasor Representation.ctl" = enum32{"(g, s)", "(m, phi)"}
  T74 = typedef "Image.lvlib/Image Save File Format.ctl" = enum16{"PNG", "JPEG", "BMP"}
  T75 = typedef "LVPointDoubleTypeDef.ctl" = cluster{"Cursor X":dbl, "Cursor Y":dbl}
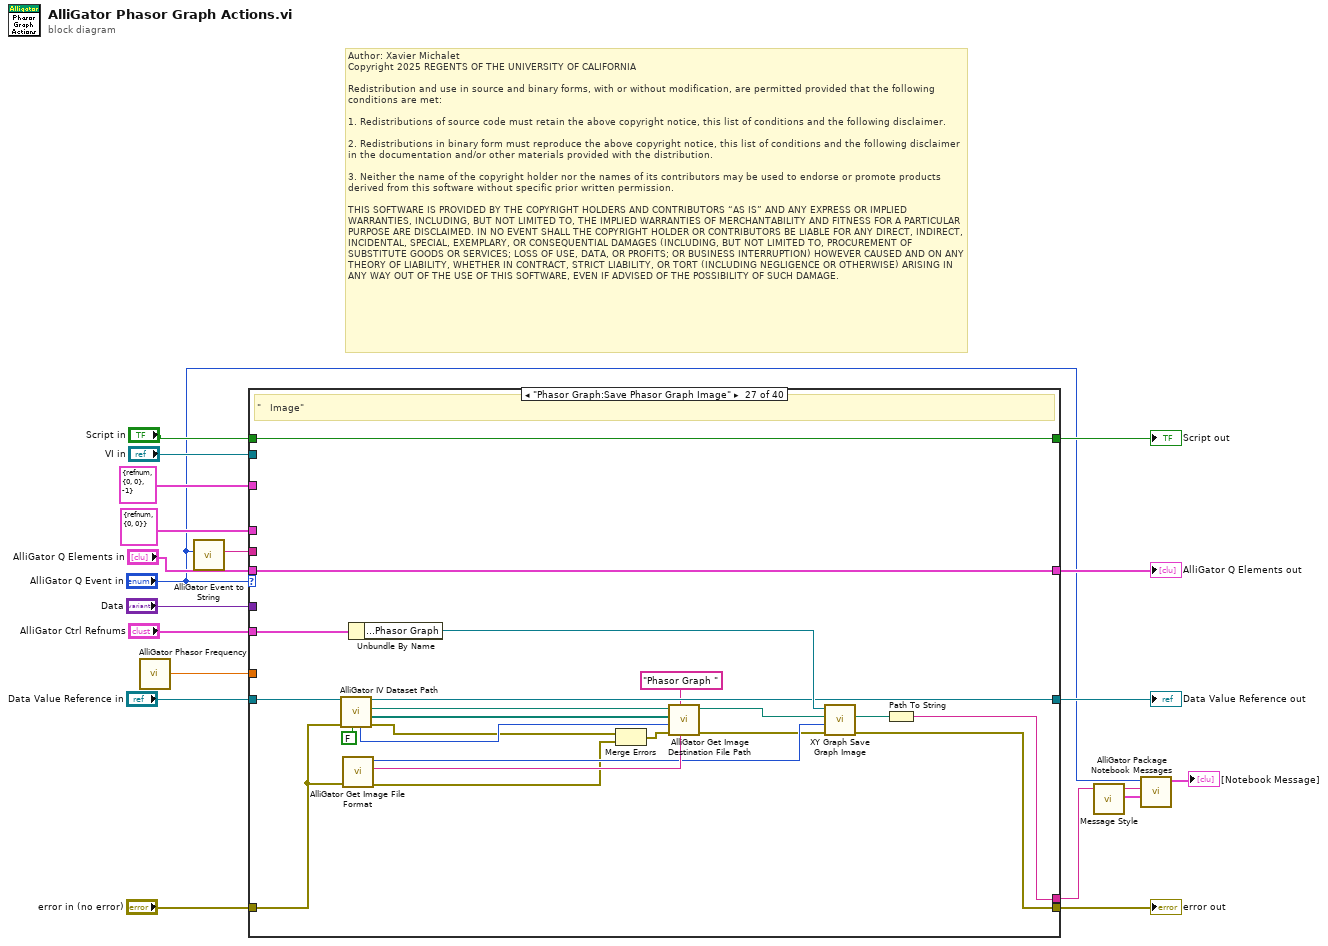
[diagram p0: block diagram]
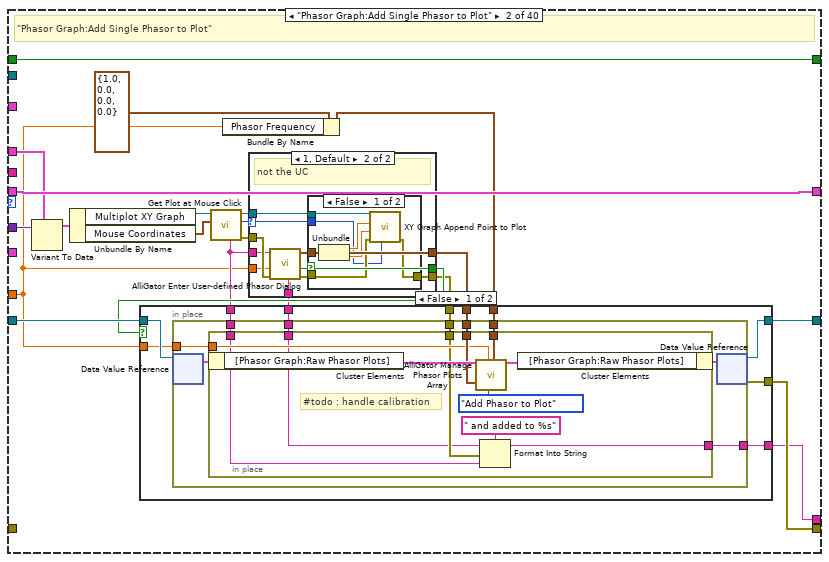
[diagram p3: hidden frame]
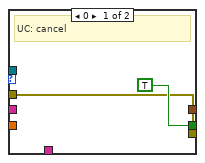
[diagram p4: hidden frame]
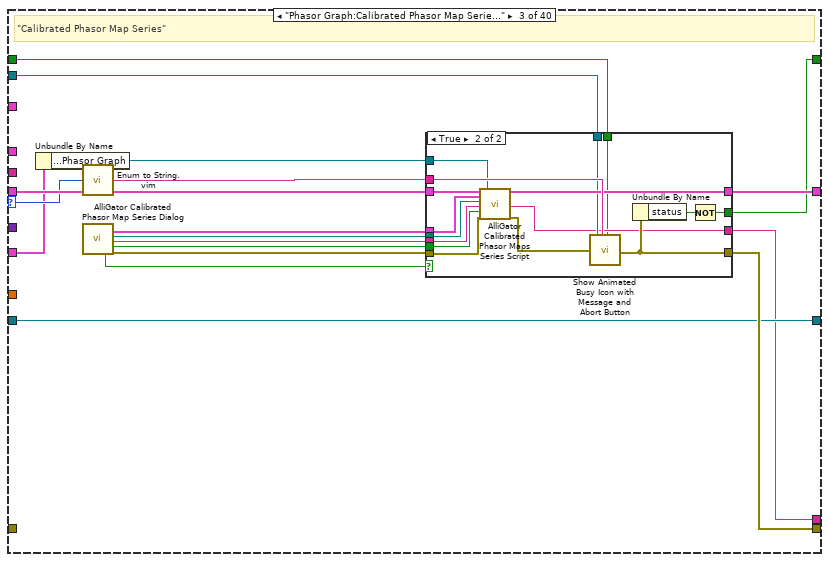
[diagram p7: hidden frame]
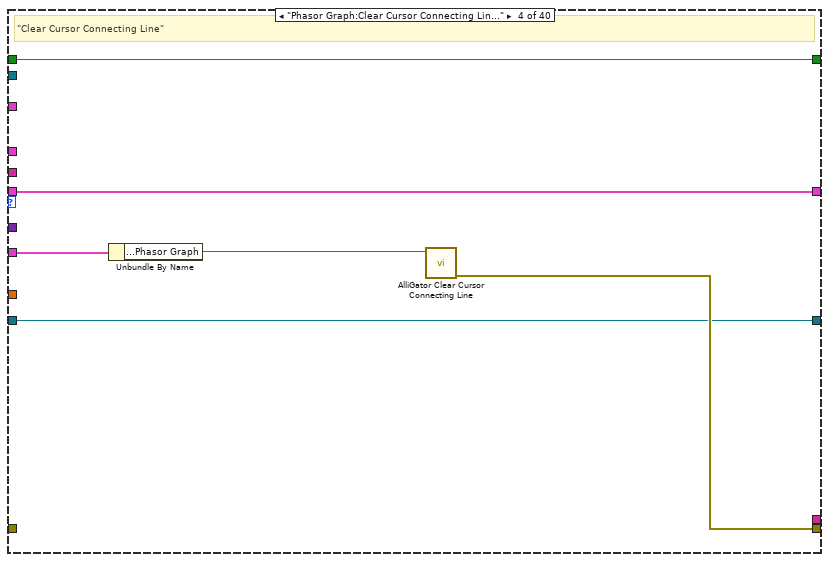
[diagram p9: hidden frame]
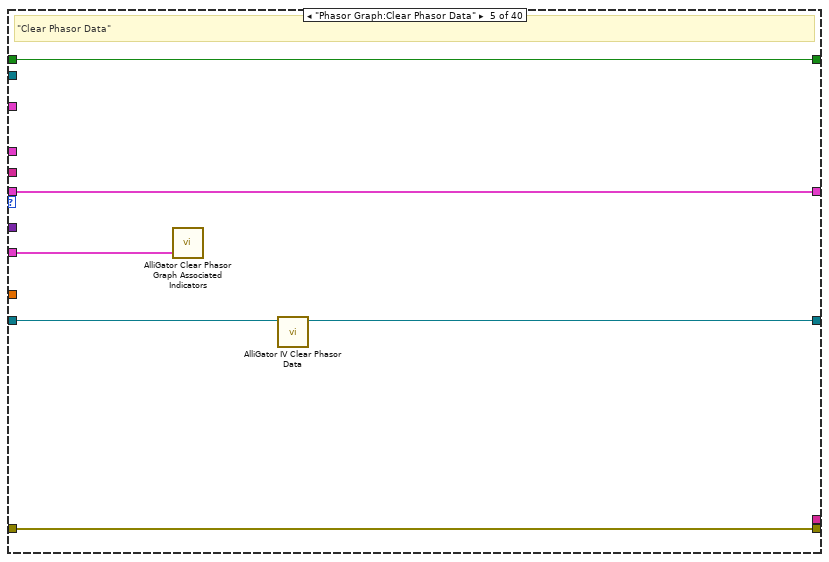
[diagram p10: hidden frame]
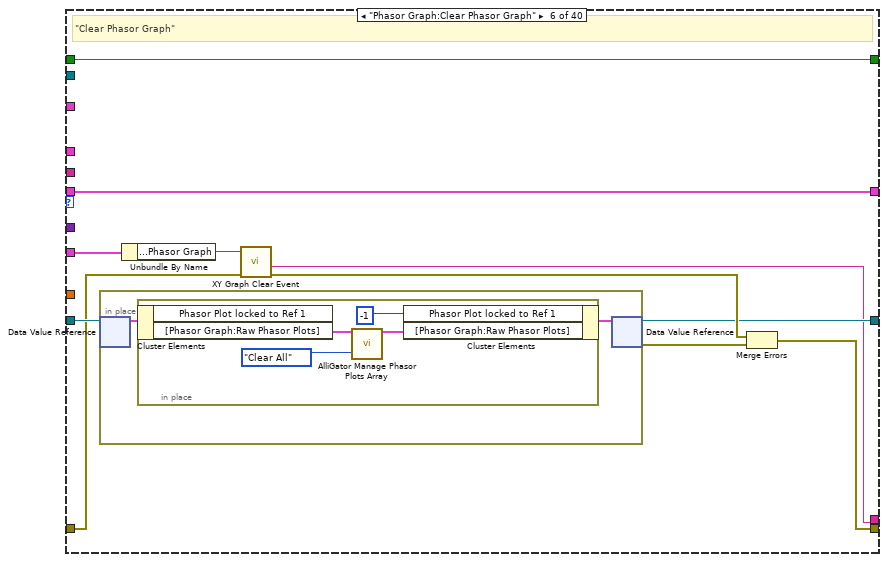
[diagram p11: hidden frame]
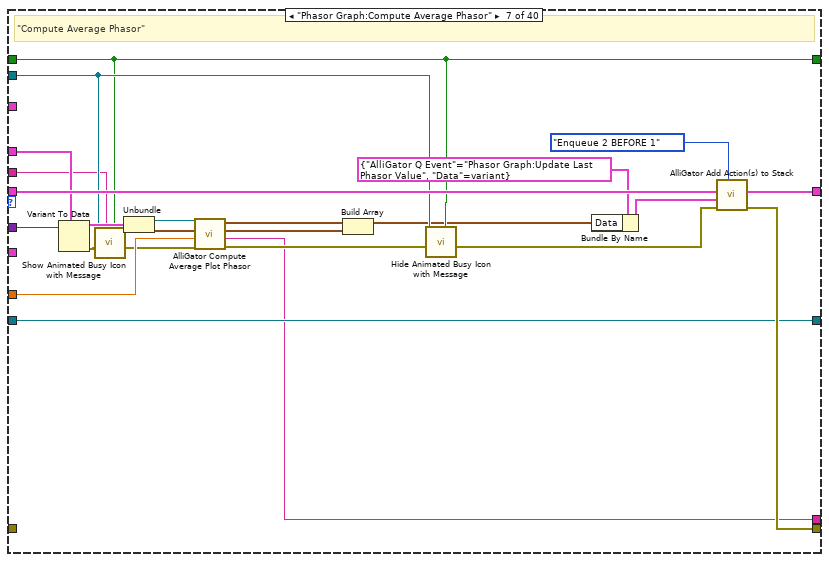
[diagram p12: hidden frame]
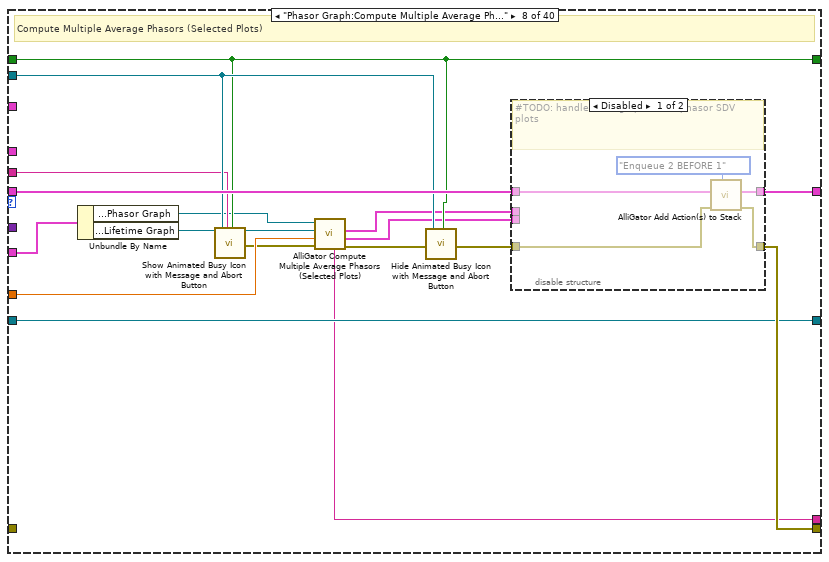
[diagram p13: hidden frame]
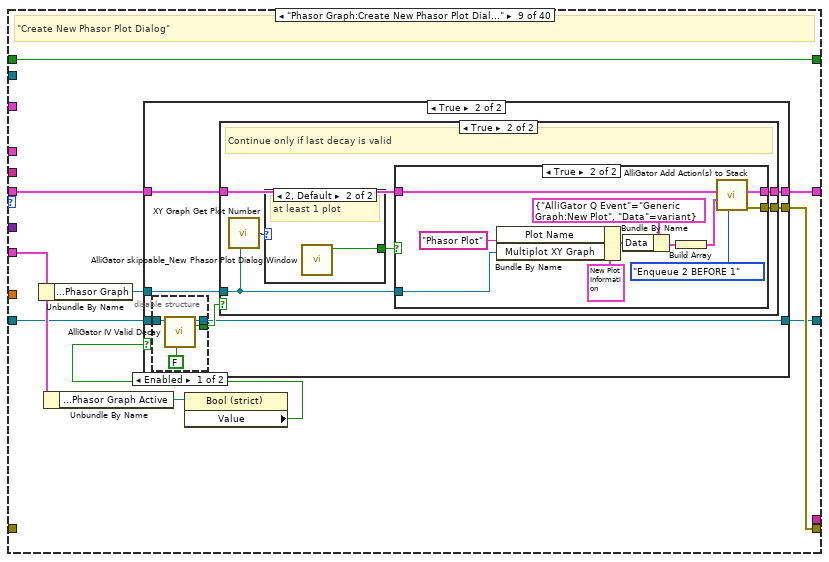
[diagram p15: hidden frame]
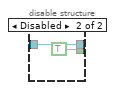
[diagram p17: hidden frame]
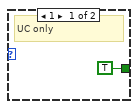
[diagram p19: hidden frame]
diagram:
  # "Author: Xavier Michalet\nCopyright 2025 REGENTS OF THE UNIVERSITY OF CALIFORNIA\n\nRedistribution and use in source and binary forms, with or without modification, are permitted provided that the following conditions are met:\n\n1. Redistributions of source code must retain the above copyright notice, this list of conditions and the following disclaimer.\n\n2. Redistributions in binary form must reproduce the above copyright notice, this list of conditions and the following disclaimer in the documentation and/or other materials provided with the distribution.\n\n3. Neither the name of the copyright holder nor the names of its contributors may be used to endorse or promote products derived from this software without specific prior written permission.\n\nTHIS SOFTWARE IS PROVIDED BY THE COPYRIGHT HOLDERS AND CONTRIBUTORS “AS IS” AND ANY EXPRESS OR IMPLIED WARRANTIES, INCLUDING, BUT NOT LIMITED TO, THE IMPLIED WARRANTIES OF MERCHANTABILITY AND FITNESS FOR A PARTICULAR PURPOSE ARE DISCLAIMED. IN NO EVENT SHALL THE COPYRIGHT HOLDER OR CONTRIBUTORS BE LIABLE FOR ANY DIRECT, INDIRECT, INCIDENTAL, SPECIAL, EXEMPLARY, OR CONSEQUENTIAL DAMAGES (INCLUDING, BUT NOT LIMITED TO, PROCUREMENT OF SUBSTITUTE GOODS OR SERVICES; LOSS OF USE, DATA, OR PROFITS; OR BUSINESS INTERRUPTION) HOWEVER CAUSED AND ON ANY THEORY OF LIABILITY, WHETHER IN CONTRACT, STRICT LIABILITY, OR TORT (INCLUDING NEGLIGENCE OR OTHERWISE) ARISING IN ANY WAY OUT OF THE USE OF THIS SOFTWARE, EVEN IF ADVISED OF THE POSSIBILITY OF SUCH DAMAGE."
  n1 = call "AlliGator Phasor Frequency.vi"() -> ("Phasor Frequency"=w14:dbl[unit])
  n2 = call "AlliGator Event to String.vi"("AlliGator Q Event"="AlliGator Q Event in") -> ("String"=w5:string)  [unwired: 8 in]
  n3 = case shown="\"Phasor Graph:Save Phasor Graph Image\"" "AlliGator Q Event in" {
    selector: "AlliGator Q Event in" -> [_ _ w113 _ _ _ _ _ _ _ _ _ _ _ _ _ _ _ _ _ _ _ _ _ _ _ _ _ _ _ _ _ _ _ _ _ _ _ _ _]
    tunnel: "Data" -> [_ w45 _ _ _ _ w187 _ _ _ _ w294 w315 w331 _ _ w453 w473 _ _ _ _ w519 w530 w545 w575 _ w627 w657 w672 w704 w739 w797 w812 _ w852 w889 w921 _ _]
    tunnel: "AlliGator Q Elements in" -> [w23 w44 w115 w140 w146 w157 w182 w204 w221 w262 w280 w296 w316 w337 w352 w381 w457 w472 w477 w481 w493 w508 w518 w529 w544 w577 w608 w628 w658 w671 w703 w726 w795 w810 w835 w851 w890 w937 w961 w966]
    tunnel: [w23 w44 w114 w140 w146 w157 w181 w203 w220 w261 w280 w296 w316 w337 w352 w380 w457 w472 w477 w481 w493 w508 w518 w529 w544 w577 w608 w628 w658 w670 w702 w725 w795 w810 w835 w850 w890 w937 w961 w965] -> w10
    tunnel: "VI in" -> [_ _ w100 _ _ _ w171 w197 _ _ _ _ _ _ _ w372 w450 _ _ _ _ _ _ _ _ _ _ _ _ _ _ _ _ _ w818 _ w856 w904 _ _]
    tunnel: w14 -> [_ w24 _ _ _ _ w176 w201 _ _ _ _ _ w334 w346 _ _ w459 _ _ _ _ _ _ _ _ _ _ _ w667 w697 _ _ _ w826 _ w859 w907 w956 _]
    tunnel: [w22 w42 w109 w139 w145 w156 w167 w195 w219 w265 w279 w295 w314 w336 w351 w371 w445 w471 w476 w480 w492 w507 w517 w528 w537 w576 w605 w618 w649 w668 w700 w734 w794 w808 w815 w842 w854 w901 w955 w964] -> w11
    tunnel: "Script in" -> [w22 w42 w112 w139 w145 w156 w167 w195 w219 w265 w279 w295 w314 w336 w351 w371 w445 w471 w476 w480 w492 w507 w517 w528 w537 w576 w605 w618 w649 w668 w700 w734 w794 w808 w815 w842 w854 w901 w955 w964]
    tunnel: "error in (no error)" -> [w21 _ _ _ w141 w147 _ _ _ w264 _ _ _ _ w344 _ _ w462 w475 w478 _ w506 _ _ _ _ w589 _ _ _ _ _ _ _ w814 _ _ _ _ _]
    tunnel: [w21 w31 w110 w137 w141 w150 w172 w198 w217 w264 w277 w293 w313 w335 w343 w379 w447 w466 w475 w478 w488 w506 w512 w523 w536 w571 w593 w616 w648 w666 w696 w733 w782 w800 w821 w841 w861 w911 w943 w963] -> w8
    tunnel: "AlliGator Ctrl Refnums" -> [_ _ w101 w136 w144 w153 _ w193 w215 _ w276 w292 _ w333 w349 w377 w451 w470 _ _ w491 _ w510 w521 _ w569 w601 _ w646 w663 _ w731 w792 w806 w820 w839 w866 w916 w948 _]
    tunnel: "Data Value Reference in" -> [w20 w40 w99 w135 w143 w152 w170 w196 w213 w263 w273 w291 w312 w329 w345 w374 w448 w460 w474 w479 w486 w505 w515 w526 w534 w568 w600 w614 w645 w664 w694 w730 w790 w803 w817 w838 w855 w903 w944 w962]
    tunnel: [w20 w41 w99 w135 w142 w151 w170 w196 w212 w263 w273 w290 w311 w329 w345 w375 w449 w468 w474 w479 w487 w505 w516 w527 w535 w567 w599 w615 w645 w664 w694 w729 w784 w804 w817 w838 w855 w903 w944 w962] -> w19
    tunnel: [_ w28 w98 _ _ w148 w169 w190 _ _ _ w283 w297 w328 _ w373 w446 w467 _ _ w485 _ w511 w522 w532 w561 w594 w609 w644 w659 w693 _ _ _ _ w836 w853 w902 _ _] -> w2
    tunnel: T17 {"Multiplot XY Graph"=refnum, "Mouse Coordinates"={"Horizontal"=0, "Vertical"=0}} ("Mouse Click Event Data") -> [_ w39 _ _ _ _ w168 _ _ _ _ _ _ _ _ _ _ _ _ _ _ _ _ _ w533 _ _ _ _ _ _ _ _ _ _ _ _ _ _ _]
    tunnel: T14 {"Multiplot XY Graph"=refnum, "Mouse Coordinates"={"Horizontal"=0, "Vertical"=0}, "Plot Index"=-1} ("Selected Plot Info") -> [_ _ _ _ _ _ _ _ _ _ _ _ _ _ _ _ _ _ _ _ _ _ _ _ _ _ _ _ _ _ _ _ _ _ _ _ _ _ _ _]
    tunnel: w5 -> [_ _ _ _ _ _ w164 w194 _ _ _ _ _ _ _ w370 w444 _ _ _ _ _ _ _ _ _ _ _ _ _ _ _ _ _ w813 _ _ _ _ _]
    frame "---- Phasor Graph ----", Default {
    }
    frame "Phasor Graph:Add Single Phasor to Plot" {
      # "\"Phasor Graph:Add Single Phasor to Plot\""
      n4 = Variant To Data(type=w39, Variant=w45) -> (data=w43:T17)  [unwired: 1 in, 1 out]
      n5 = Unbundle By Name(w43) -> ("Multiplot XY Graph"=w38:T15, "Mouse Coordinates"=w37:T16)
      n6 = call-poly "Get Plot at Mouse Click.vi"("Mouse Click Coordinates"=w37, "XYGraph Ref"=w38) -> ("error out"=w36:errorcluster, "Plot at Coordinates"=w33:i32, "XYGraph Ref"=w27:T15, "Plot Name"=w29:string)  [unwired: 3 in, 3 out]
      n7 = Bundle By Name(cluster=T18 {"m"=1.0, "phi"=0.0, "Phasor Frequency"=0.0, "Reference Lifetime"=0.0} ("Calibration Phasor"), "Phasor Frequency"=w24) -> (w25:T18)
      n8 = case shown="1, Default" w33 {
        selector: w33 -> [_ w49]
        tunnel: w36 -> [w46 w57]
        tunnel: w29 -> [_ w56]
        tunnel: w24 -> [_ w55]
        tunnel: [_ w52] -> w35
        tunnel: [TRUE ("Cancelled?") w48] -> w34
        tunnel: [_ w54] -> w32
        tunnel: [w46 w50] -> w30
        tunnel: w27 -> [_ w53]
        frame 0 {
          # "UC: cancel"
        }
        frame 1, Default {
          # "not the UC"
          n9 = call "AlliGator Enter User-defined Phasor Dialog.vi"("Error In"=w57, "Phasor Frequency"=w55, "Phasor Plot Name"=w56) -> ("Error Out"=w51:errorcluster, "Cancelled?"=w48:bool, "New Phasor (g, s)"=w52:T29, "Message"=w54:string)  [unwired: 5 in]
          n10 = case shown="False" w48 {
            tunnel: w53 -> [w64 _]
            tunnel: w52 -> [w63 _]
            tunnel: w51 -> [w60 w65]
            tunnel: [w59 w65] -> w50
            tunnel: w49 -> [w58 _]
            frame False {
              n11 = Unbundle(w63) -> ("g"=w62:dbl, "s"=w61:dbl)
              n12 = call "XY Graph Append Point to Plot.vi"("Plot ID (-1: last)"=w58, "error in (no error)"=w60, "y"=w61, "x"=w62, "XYGraph in"=w64) -> ("error out"=w59:errorcluster)  [unwired: 3 in, 3 out]
            }
            frame True {
            }
          }
        }
      }
      n13 = case shown="False" w34 {
        tunnel: w40 -> [w75 w97]
        tunnel: [w74 w97] -> w41
        tunnel: w35 -> [w73 _]
        tunnel: w32 -> [w69 _]
        tunnel: w24 -> [w72 _]
        tunnel: [w71 w96] -> w31
        tunnel: w30 -> [w70 w96]
        tunnel: w29 -> [w68 _]
        tunnel: [w67 _] -> w28
        tunnel: w25 -> [w66 _]
        frame False {
          n14 = in-place {
            in-place-border: w73 -> [w82]
            in-place-border: w72 -> [w81]
            in-place-border: w70 -> [w80]
            in-place-border: w69 -> [w79]
            in-place-border: w68 -> [w78]
            in-place-border: [w77] -> w67
            in-place-border: w66 -> [w76]
            n15 = in-place-dvr #1(w75) -> (w84:T33)  [unwired: 1 out]
            n16 = in-place {
              in-place-border: w82 -> [w92]
              in-place-border: w81 -> [w91]
              in-place-border: w80 -> [w90]
              in-place-border: w79 -> [w89]
              in-place-border: w78 -> [w87]
              in-place-border: [w86] -> w77
              in-place-border: w76 -> [w85]
              # "#todo : handle calibration"
              n17 = in-place-cluster #2(w84) -> ("[Phasor Graph:Raw Phasor Plots]"=w93:T51[])
              n18 = call "AlliGator Manage Phasor Plots Array.vi"("[Raw Phasor Plot] in"=w93, "Raw Phasor (g, s)"=w92, "Phasor Frequency"=w91, "[Raw Phasor Plot] Action"=AlliGator_Raw_Phasor_Plot_Array_Action."Add Phasor to Plot", "Calibration Phasor"=w85) -> ("[Raw Phasor Plot] out"=w95:T51[])  [unwired: 14 in]
              n19 = Format Into String(format string=" and added to %s", initial string=w89, error in=w90, w87) -> (resulting string=w86:string)  [unwired: 1 out]
              n20 = in-place-cluster #2("[Phasor Graph:Raw Phasor Plots]"=w95) -> (w83:T33)
            }
            n21 = in-place-dvr #1(w83) -> (w74:refnum<data-value>, w71:errorcluster)
          }
        }
        frame True {
        }
      }
    }
    frame "Phasor Graph:Calibrated Phasor Map Series" {
      # "\"Calibrated Phasor Map Series\""
      n22 = Unbundle By Name(w101) -> ("Registered Events Ctrl Refnums.Phasor Graph"=w102:refnum<vi>)
      n23 = call "Enum to String.vim"("Enum"=w113) -> ("String"=w111:string)
      n24 = call "AlliGator Calibrated Phasor Map Series Dialog.vi"() -> ("OK"=w103:bool, "Calibration Map/Gate Step List"=w107:T68[], "Destination Folder"=w106:path, "File Suffix (# Steps will be added)"=w105:string, "Save Phasor Plot"=w104:bool, "error out"=w108:errorcluster)  [unwired: 14 in]
      n25 = case shown="True" w103 {
        tunnel: w115 -> [w118 w130]
        tunnel: [w118 w129] -> w114
        tunnel: w108 -> [w117 w127]
        tunnel: w102 -> [_ w128]
        tunnel: w112 -> [w116 w119]
        tunnel: w111 -> [_ w134]
        tunnel: [w117 w133] -> w110
        tunnel: [w116 w131] -> w109
        tunnel: w107 -> [_ w126]
        tunnel: w106 -> [_ w125]
        tunnel: w105 -> [_ w124]
        tunnel: w104 -> [_ w123]
        tunnel: w100 -> [_ w121]
        tunnel: [_ w120] -> w98
        frame False {
        }
        frame True {
          n26 = call "AlliGator Calibrated Phasor Maps Series Script.vi"("Alligator Queue Elements in"=w130, "Calibration Map/Gate Step List"=w126, "Destination Folder"=w125, "File Suffix (# Steps will be added)"=w124, "Save Phasor Plot"=w123, "Error In"=w127, "Phasor Graph refnum"=w128) -> ("Alligator Queue Elements out"=w129:T4[], "Message"=w120:string, "Error Out"=w122:errorcluster)  [unwired: 10 in]
          n27 = call "Show Animated Busy Icon with Message and Abort Button.vi"("Already active? (F)"=w119, "Message"=w134, "Target VI reference"=w121, "Error In"=w122) -> ("Error Out"=w133:errorcluster)  [unwired: 15 in]
          n28 = Unbundle By Name(w133) -> ("status"=w132:bool)
          n29 = Not(x=w132) -> (.not. x?=w131:bool)
        }
      }
    }
    frame "Phasor Graph:Clear Cursor Connecting Line" {
      # "\"Clear Cursor Connecting Line\""
      n30 = Unbundle By Name(w136) -> ("Registered Events Ctrl Refnums.Phasor Graph"=w138:refnum<vi>)
      n31 = call "AlliGator Clear Cursor Connecting Line.vi"("Phasor Graph Refnum"=w138) -> ("Error Out"=w137:errorcluster)  [unwired: 10 in]
    }
    frame "Phasor Graph:Clear Phasor Data" {
      # "\"Clear Phasor Data\""
      n32 = call "AlliGator Clear Phasor Graph Associated Indicators.vi"("AlliGator Ctrl Refnums"=w144) -> ()  [unwired: 11 in]
      n33 = call "AlliGator IV Clear Phasor Data.vi"("Data Value Reference in"=w143) -> ("Data Value Reference out"=w142:refnum<data-value>)  [unwired: 10 in]
    }
    frame "Phasor Graph:Clear Phasor Graph" {
      # "\"Clear Phasor Graph\""
      n34 = in-place {
        n35 = in-place-dvr #3(w152) -> (w159:T33)  [unwired: 1 out]
        n36 = in-place {
          n37 = in-place-cluster #4(w159) -> ("[Phasor Graph:Raw Phasor Plots]"=w163:T51[])  [unwired: 1 out]
          n38 = call "AlliGator Manage Phasor Plots Array.vi"("[Raw Phasor Plot] in"=w163, "[Raw Phasor Plot] Action"=AlliGator_Raw_Phasor_Plot_Array_Action."Clear All") -> ("[Raw Phasor Plot] out"=w162:T51[])  [unwired: 17 in]
          n39 = in-place-cluster #4("Phasor Plot locked to Ref 1"=-1 ("Plot at Coordinates"), "[Phasor Graph:Raw Phasor Plots]"=w162) -> (w158:T33)
        }
        n40 = in-place-dvr #3(w158) -> (w151:refnum<data-value>, w149:errorcluster)
      }
      n41 = Unbundle By Name(w153) -> ("Registered Events Ctrl Refnums.Phasor Graph"=w155:refnum<vi>)
      n42 = call "XY Graph Clear Event.vi"("Error In"=w147, "XYGraph Ref"=w155) -> ("Error Out"=w154:errorcluster, "Message"=w148:string)  [unwired: 7 in, 1 out]
      n43 = Merge Errors(w154, w149) -> (w150:errorcluster)
    }
    frame "Phasor Graph:Compute Average Phasor" {
      # "\"Compute Average Phasor\""
      n44 = Variant To Data(type=w168, Variant=w187) -> (data=w183:T17, error out=w186:errorcluster)  [unwired: 1 in]
      n45 = call "Show Animated Busy Icon with Message.vi"("Already active? (F)"=w167, "Message"=w164, "Error In"=w186, "Target VI Refnum"=w171) -> ("Error Out"=w175:errorcluster)  [unwired: 7 in]
      n46 = Unbundle(w183) -> ("Multiplot XY Graph"=w185:T15, "Mouse Coordinates"=w184:T16)
      n47 = call "AlliGator Compute Average Plot Phasor.vi"("error in (no error)"=w175, "Phasor Frequency"=w176, "Mouse Click Coordinates"=w184, "XYGraph Ref"=w185) -> ("error out"=w177:errorcluster, "Result String"=w169:string, "Phasor SDV (g, s)"=w165:T29, "Phasor (g, s)"=w174:T29)  [unwired: 4 in]
      n48 = Build Array(w174, w165) -> (w166:T29[])
      n49 = call "Hide Animated Busy Icon with Message.vi"("Already active? (F)"=w167, "Error In"=w177, "Target VI reference"=w171) -> ("Error Out"=w173:errorcluster)  [unwired: 8 in]
      n50 = Bundle By Name(cluster=T4 {"AlliGator Q Event"=enum."Phasor Graph:Update Last Phasor Value", "Data"=variant} ("Alligator Atomic Action"), "Data"=w166) -> (w179:T4)
      n51 = call-poly "AlliGator Add Action(s) to Stack.vi"("Elements Order in Action Stack (Default: 2 BEFORE 1)"=Alligator_Elements_Order_in_Action_Stack."Enqueue 2 BEFORE 1", "Error In"=w173, "Alligator Atomic Action"=w179, "Alligator Queue Element 1"=w182) -> ("Error Out"=w172:errorcluster, "Alligator Queue Element 1 (+ 2)"=w181:T4[])  [unwired: 6 in]
    }
    frame "Phasor Graph:Compute Multiple Average Phasors (Selected Plots)" {
      # "Compute Multiple Average Phasors (Selected Plots)"
      n52 = Unbundle By Name(w193) -> ("Registered Events Ctrl Refnums.Phasor Graph"=w192:refnum<vi>, "Registered Events Ctrl Refnums.Lifetime Graph"=w191:refnum<vi>)
      n53 = call "Show Animated Busy Icon with Message and Abort Button.vi"("Already active? (F)"=w195, "Message"=w194, "Target VI reference"=w197) -> ("Error Out"=w200:errorcluster)  [unwired: 16 in]
      n54 = call "AlliGator Compute Multiple Average Phasors (Selected Plots).vi"("error in (no error)"=w200, "Phasor Frequency"=w201, "Lifetime Graph Ref"=w191, "Phasor Graph Ref"=w192) -> ("error out"=w202:errorcluster, "Phasor SDV Plot"=w188:cluster{"Array":dbl[], "Array":dbl[]}, "Average Phasor Plot"=w189:cluster{"Array":dbl[], "Array":dbl[]}, "Result String"=w190:string)  [unwired: 4 in]
      n55 = call "Hide Animated Busy Icon with Message and Abort Button.vi"("Already active? (F)"=w195, "Target VI reference"=w197, "Error In"=w202) -> ("Error Out"=w199:errorcluster)  [unwired: 16 in]
      n56 = disable-structure shown="Disabled" {
        disable-tunnel: w204 -> [w209 w211]
        disable-tunnel: [w208 w211] -> w203
        disable-tunnel: w199 -> [w206 w210]
        disable-tunnel: [w205 w210] -> w198
        disable-tunnel: w189 -> [_ _]
        disable-tunnel: w188 -> [_ _]
        frame Disabled {
          # "#TODO: handle average phasor & phasor SDV plots"
          n57 = call-poly "AlliGator Add Action(s) to Stack.vi"("Elements Order in Action Stack (Default: 2 BEFORE 1)"=Alligator_Elements_Order_in_Action_Stack."Enqueue 2 BEFORE 1", "Error In"=w206, "Alligator Queue Element 1"=w209) -> ("Error Out"=w205:errorcluster, "Alligator Queue Element 1 (+ 2)"=w208:T4[])  [unwired: 7 in]
        }
        frame Enabled {
        }
      }
    }
    frame "Phasor Graph:Create New Phasor Plot Dialog" {
      # "\"Create New Phasor Plot Dialog\""
      n58 = Unbundle By Name(w215) -> ("Registered Events Ctrl Refnums.Phasor Graph"=w218:refnum<vi>)
      n59 = Unbundle By Name(w215) -> ("Phasor Graph Ctrl Refnums.Phasor Graph Active"=w216:refnum<vi>)
      n60 = property class="Bool (strict)"(reference=w216) -> ("Value"=w214:bool)  [unwired: 1 in, 2 out]
      n61 = case shown="True" w214 {
        tunnel: w221 -> [w223 w230]
        tunnel: [w223 w229] -> w220
        tunnel: w218 -> [_ w228]
        tunnel: [_ w227] -> w217
        tunnel: w213 -> [w222 w226]
        tunnel: [w222 w224] -> w212
        frame False {
        }
        frame True {
          n62 = disable-structure shown="Enabled" {
            disable-tunnel: w226 -> [w234 w236]
            disable-tunnel: [w232 TRUE ("Valid Decay")] -> w225
            disable-tunnel: [w231 w236] -> w224
            frame Enabled {
              n63 = call "AlliGator IV Valid Decay.vi"("Get (F)/ Set (T)"=FALSE, "AlliGator IV DVR in"=w234) -> ("Valid Decay"=w232:bool, "AlliGator IV DVR out"=w231:refnum<data-value>)  [unwired: 7 in, 1 out]
            }
            frame Disabled {
            }
          }
          n64 = case shown="True" w225 {
            tunnel: w230 -> [w237 w243]
            tunnel: [w237 w242] -> w229
            tunnel: w228 -> [_ w239]
            tunnel: [_ w238] -> w227
            frame False {
              # "Last decay invalid"
            }
            frame True {
              # "Continue only if last decay is valid"
              n65 = call "XY Graph Get Plot Number.vi"("XYGraph"=w239) -> ("# Plots"=w240:i32)  [unwired: 8 in]
              n66 = case shown="2, Default" w240 {
                tunnel: [TRUE ("T button?") w245] -> w241
                frame 1 {
                  # "UC only"
                }
                frame 2, Default {
                  # "at least 1 plot"
                  n67 = call "AlliGator skippable_New Phasor Plot Dialog Window.vi"() -> ("New Plot?"=w245:bool)  [unwired: 10 in, 1 out]
                }
              }
              n68 = case shown="True" w241 {
                tunnel: w243 -> [w246 w257]
                tunnel: [w246 w256] -> w242
                tunnel: w239 -> [_ w252]
                tunnel: [_ w251] -> w238
                frame False {
                }
                frame True {
                  n69 = Bundle By Name(cluster=T21 {"Multiplot XY Graph"=refnum, "Plot Name"="", "Plot Scales"={"X Scale"=0, "Y Scale"=0}, "Plot Interpolation"=0, "Point Style"=enum."Empty Square", "Plot Color"=15781887, "Plot Metadata"=variant} ("New Plot Information"), "Plot Name"="Phasor Plot", "Multiplot XY Graph"=w252) -> (w250:T21)
                  n70 = Bundle By Name(cluster=T4 {"AlliGator Q Event"=enum."Generic Graph:New Plot", "Data"=variant} ("Alligator Atomic Action"), "Data"=w250) -> (w248:T4)
                  n71 = Build Array(w248) -> (w254:T4[])
                  n72 = call-poly "AlliGator Add Action(s) to Stack.vi"("Elements Order in Action Stack (Default: 2 BEFORE 1)"=Alligator_Elements_Order_in_Action_Stack."Enqueue 2 BEFORE 1", "Alligator Queue Element 2"=w254, "Alligator Queue Element 1"=w257) -> ("Error Out"=w251:errorcluster, "Alligator Queue Element 1 (+ 2)"=w256:T4[])  [unwired: 7 in]
                }
              }
            }
          }
        }
      }
    }
    frame "Phasor Graph:Cursor Move" {
      # "\"Phasor Graph:Cursor Move\""
      n73 = call "Alligator Variables Storage.vi"("AlliGator Variable"=AlliGator_Variables_List."Phasor Graph:Show Line") -> ("Data out"=w259:variant)  [unwired: 8 in, 2 out]
      n74 = call-poly "Variant to Data.vi"("Variant"=w259) -> ("Value"=w258:bool)  [unwired: 8 in]
      n75 = case shown="True" w258 {
        tunnel: w262 -> [w266 w270]
        tunnel: [w266 w268] -> w261
        frame False {
        }
        frame True {
          n76 = Build Array(T4 {"AlliGator Q Event"=enum."Phasor Graph:Draw Cursor Connecting Line", "Data"=variant} ("Time-Gated Phasor Q Element"), T4 {"AlliGator Q Event"=enum."Phasor Graph:Find UC Intersection", "Data"=variant} ("Time-Gated Phasor Q Element")) -> (w269:T4[])
          n77 = call-poly "AlliGator Add Action(s) to Stack.vi"("Elements Order in Action Stack (Default: 2 BEFORE 1)"=Alligator_Elements_Order_in_Action_Stack."Enqueue 2 AFTER 1", "Alligator Queue Element 2"=w269, "Alligator Queue Element 1"=w270) -> ("Alligator Queue Element 1 (+ 2)"=w268:T4[])  [unwired: 7 in, 1 out]
        }
      }
    }
    frame "Phasor Graph:Draw Cursor Connecting Line" {
      # "\"Draw Cursor Connecting Line\""
      n78 = Unbundle By Name(w276) -> ("Phasor Graph Ctrl Refnums.Show Line"=w275:refnum<vi>, "Registered Events Ctrl Refnums.Phasor Graph"=w278:refnum<vi>)
      n79 = property class="Bool (strict)"(reference=w275) -> ("Value"=w274:bool)  [unwired: 1 in, 2 out]
      n80 = case shown="True" w274 {
        tunnel: w278 -> [_ w282]
        tunnel: [_ w281] -> w277
        frame False {
        }
        frame True {
          n81 = call "AlliGator Draw Cursor Connecting Line.vi"("Phasor Graph Refnum"=w282) -> ("Error Out"=w281:errorcluster)  [unwired: 10 in]
        }
      }
    }
    frame "Phasor Graph:Export Selected Phasor Plots Data" {
      w288 = TRUE  # Save as...
      # "\"Export Selected Phasor Plots Data\""
      n82 = call-poly "Variant to Data.vi"("Variant"=w294) -> ("Value"=w287:bool)  [unwired: 8 in]
      n83 = Unbundle By Name(w292) -> ("Registered Events Ctrl Refnums.Phasor Graph"=w289:refnum<vi>)
      n84 = call "AlliGator IV [Raw Phasor Plot].vi"("Get (F)/ Set (T)"=FALSE, "AlliGator IV DVR in"=w291) -> ("error out"=w285:errorcluster, "[Raw Phasor Plots]"=w286:T51[], "AlliGator IV DVR out"=w290:refnum<data-value>)  [unwired: 7 in]
      n85 = call "AlliGator Save Multiple Phasor Plots Additional Data.vi"("Save as..."=w288, "error in (no error)"=w285, "Raw Phasor Plots"=w286, "All Plots"=w287, "Phasor Graph"=w289) -> ("Error Out"=w293:errorcluster, "Message"=w283:string)  [unwired: 5 in]
    }
    frame "Phasor Graph:Export Single Phasor Plot Data" {
      # "\"Export Single Phasor Plot Data\""
      n86 = Variant To Data(type=T26 {"Mouse Click Event Data"={"Multiplot XY Graph"=refnum, "Mouse Coordinates"={"Horizontal"=0, "Vertical"=0}}, "Save as..."=FALSE} ("output cluster"), Variant=w315) -> (data=w310:T26, error out=w299:errorcluster)  [unwired: 1 in]
      n87 = Unbundle(w310) -> ("Mouse Click Event Data"=w309:T17, "Save as..."=w303:bool)
      n88 = call "AlliGator IV [Raw Phasor Plot].vi"("Get (F)/ Set (T)"=FALSE, "error in (no error)"=w299, "AlliGator IV DVR in"=w312) -> ("error out"=w298:errorcluster, "[Raw Phasor Plots]"=w301:T51[], "AlliGator IV DVR out"=w311:refnum<data-value>)  [unwired: 6 in]
      n89 = Unbundle(w309) -> ("Multiplot XY Graph"=w305:T15, "Mouse Coordinates"=w304:T16)
      n90 = call-poly "Get Plot at Mouse Click.vi"("error in (no error)"=w298, "Mouse Click Coordinates"=w304, "XYGraph Ref"=w305) -> ("error out"=w308:errorcluster, "Plot at Coordinates"=w302:i32, "XYGraph Ref"=w307:T15)  [unwired: 2 in, 4 out]
      n91 = case shown="1, Default" w302 {
        selector: w302 -> [_ w321]
        tunnel: w308 -> [w317 w326]
        tunnel: w307 -> [_ w327]
        tunnel: w303 -> [_ w325]
        tunnel: w301 -> [_ w323]
        tunnel: [w317 w319] -> w313
        tunnel: [_ w318] -> w297
        frame -1, 0 {
          # "UC or not found"
        }
        frame 1, Default {
          n92 = call "AlliGator IV Script Destination File Path.vi"() -> ("Destination File Path"=w320:path)
          n93 = Decrement(x=w321) -> (x-1=w324:i32)
          n94 = Index Array(array=w323, index=w324) -> (element=w322:T51)
          n95 = call "AlliGator Save Phasor Plot Additional Data.vi"("Save as..."=w325, "Phasor Plot Folder Path (empty)"=w320, "error in (no error)"=w326, "Raw Phasor Plot"=w322, "Selected Plot"=w321, "Phasor Graph"=w327) -> ("Error Out"=w319:errorcluster, "Message"=w318:string)  [unwired: 4 in]
        }
      }
    }
    frame "Phasor Graph:Export Single Phasor Plot Phase Lifetimes" {
      # "\"Export Single Phasor Plot Phase Lifetime\""
      n96 = Unbundle By Name(w333) -> ("Registered Events Ctrl Refnums.Phasor Graph"=w332:refnum<vi>)
      n97 = call-poly "Variant to Data.vi"("Variant"=w331) -> ("Path"=w330:path)  [unwired: 8 in]
      n98 = call "AlliGator Export Single Phasor Plot Phase Lifetimes.vi"("Frequency"=w334, "File Path in (empty: dialog)"=w330, "Phasor Graph"=w332) -> ("Error Out"=w335:errorcluster, "Message"=w328:string)  [unwired: 6 in, 1 out]
    }
    frame "Phasor Graph:Find UC Intersection" {
      # "\"Find UC Intersection\""
      n99 = Unbundle By Name(w349) -> ("Phasor Graph Ctrl Refnums.Phasor Reference 1 Control"=w340:refnum<vi>, "Phasor Graph Ctrl Refnums.Phasor Reference 2 Control"=w339:refnum<vi>, "Registered Events Ctrl Refnums.Phasor Graph"=w350:refnum<vi>, "Phasor Graph Ctrl Refnums.Phase Lifetime 1"=w348:refnum<vi>, "Phasor Graph Ctrl Refnums.Phase Lifetime 2"=w347:refnum<vi>)
      n100 = property class="Scroll (strict)"(reference=w340) -> ("Visible"=w342:bool)  [unwired: 1 in, 2 out]
      n101 = property class="Scroll (strict)"(reference=w339) -> ("Visible"=w341:bool)  [unwired: 1 in, 2 out]
      n102 = Or(x=w342, y=w341) -> (x .or. y?=w338:bool)
      n103 = case shown="True" w338 {
        tunnel: w350 -> [_ w368]
        tunnel: w348 -> [_ w367]
        tunnel: w347 -> [_ w366]
        tunnel: w346 -> [_ w363]
        tunnel: w344 -> [w353 w360]
        tunnel: [w353 w354] -> w343
        frame False {
        }
        frame True {
          w361 = TRUE ("Visible")
          n104 = call "AlliGator Find Cursor Connecting Line Intersection(s) with Universal Circle.vi"("Error In"=w360, "XY Graph Refnum"=w368) -> ("Error Out"=w358:errorcluster, "Intersection 2"=w364:cluster{"x":dbl, "y":dbl}, "Intersection 1"=w369:cluster{"x":dbl, "y":dbl})  [unwired: 7 in]
          n105 = call "Phasor Convert (g,s,f) to (tf, tm).vi"("Error In"=w358, "Phasor Harmonic Frequency"=w363, "Phasor (g, s)"=w369) -> ("Error Out"=w359:errorcluster, "Phase Lifetime"=w365:dbl[unit])  [unwired: 6 in, 1 out]
          n106 = call "Phasor Convert (g,s,f) to (tf, tm).vi"("Error In"=w358, "Phasor Harmonic Frequency"=w363, "Phasor (g, s)"=w364) -> ("Error Out"=w357:errorcluster, "Phase Lifetime"=w362:dbl[unit])  [unwired: 6 in, 1 out]
          n107 = property class="DigNum (strict)"(reference=w367, error in=w359, "Value"=w365, "Visible"=w361) -> (error out=w356:errorcluster)  [unwired: 1 out]
          n108 = property class="DigNum (strict)"(reference=w366, error in=w357, "Value"=w362, "Visible"=w361) -> (error out=w355:errorcluster)  [unwired: 1 out]
          n109 = Merge Errors(w356, w355) -> (w354:errorcluster)
        }
      }
    }
    frame "Phasor Graph:Get Phasor Value" {
      # "\"Get Phasor Value\""
      n110 = Unbundle By Name(w377) -> ("Phasor Graph Ctrl Refnums.Phasor Graph Active"=w378:refnum<vi>)
      n111 = property class="Bool (strict)"(reference=w378) -> ("Value"=w376:bool)  [unwired: 1 in, 2 out]
      n112 = case shown="True" w376 {
        tunnel: w381 -> [w383 w399]
        tunnel: [w383 w398] -> w380
        tunnel: [_ w392] -> w379
        tunnel: w377 -> [_ w394]
        tunnel: [w382 w393] -> w375
        tunnel: w374 -> [w382 w391]
        tunnel: [_ w387] -> w373
        tunnel: w372 -> [_ w386]
        tunnel: w371 -> [_ w385]
        tunnel: w370 -> [_ w384]
        frame False {
        }
        frame True {
          n113 = Unbundle By Name(w394) -> ("Phasor Graph Ctrl Refnums.Save Phasor Graph"=w396:refnum<vi>, "Registered Events Ctrl Refnums.Phasor Graph"=w397:refnum<vi>, "Phasor Graph Ctrl Refnums.Single Step Phasor"=w389:refnum<vi>, "Phasor Graph Ctrl Refnums.Phasor Frame Slide"=w395:refnum<vi>)
          n114 = disable-structure shown="Enabled" {
            disable-tunnel: w391 -> [w403 w405]
            disable-tunnel: [w402 w405] -> w390
            disable-tunnel: [w400 TRUE ("Valid Decay")] -> w388
            frame Enabled {
              n115 = call "AlliGator IV Valid Decay.vi"("Get (F)/ Set (T)"=FALSE, "AlliGator IV DVR in"=w403) -> ("Valid Decay"=w400:bool, "AlliGator IV DVR out"=w402:refnum<data-value>)  [unwired: 7 in, 1 out]
            }
            frame Disabled {
            }
          }
          n116 = case shown="True" w388 {
            tunnel: w399 -> [w407 w438]
            tunnel: [w407 w437] -> w398
            tunnel: w397 -> [_ w418]
            tunnel: w396 -> [_ w432]
            tunnel: w395 -> [_ w430]
            tunnel: [w406 w419] -> w393
            tunnel: [_ w424] -> w392
            tunnel: w390 -> [w406 w421]
            tunnel: w389 -> [_ w417]
            tunnel: [_ w415] -> w387
            tunnel: w386 -> [_ w410]
            tunnel: w385 -> [_ w409]
            tunnel: w384 -> [_ w408]
            frame False {
            }
            frame True {
              n117 = call "AlliGator IV Dataset Path.vi"("Get (F)/ Set (T)"=FALSE, "AlliGator IV DVR in"=w421) -> ("error out"=w427:errorcluster, "AlliGator IV DVR out"=w420:refnum<data-value>, "Current Dataset"=w426:i32)  [unwired: 5 in, 2 out]
              n118 = property class="Bool (strict)"(reference=w432) -> ("Value"=w431:bool)  [unwired: 1 in, 2 out]
              n119 = Increment(x=w426) -> (x+1=w429:i32)
              n120 = call "Show Animated Busy Icon with Message.vi"("Already active? (F)"=w409, "Message"=w408, "Error In"=w427, "Target VI Refnum"=w410) -> ("Error Out"=w412:errorcluster)  [unwired: 7 in]
              n121 = call "AlliGator Get Phasor Value from Decay.vi"("Error In"=w412, "Single Step Phasor"=w417, "Phasor Graph in"=w418, "AlliGator Internal Variables DVR"=w420) -> ("Error Out"=w423:errorcluster, "Calibrated Phasor SDV"=w413:T29, "Calibrated Phasor"=w416:T29, "AlliGator Internal Variables DVR"=w419:refnum<data-value>, "Message"=w415:string)  [unwired: 2 in, 1 out]
              n122 = Build Array(w416, w413) -> (w414:T29[])
              n123 = property class="Slide (strict)"(reference=w430, error in=w423, "Scale.Maximum"=w429, "Scale.Minimum"=1.0 ("Scale.Range:Maximum"), "Value"=w429) -> (error out=w422:errorcluster)  [unwired: 1 out]
              n124 = Bundle By Name(cluster=T4 {"AlliGator Q Event"=enum."Phasor Graph:Update Last Phasor Value", "Data"=variant} ("Alligator Atomic Action"), "Data"=w414) -> (w434:T4)
              n125 = case shown="True" w431 {
                tunnel: w434 -> [w440 w442]
                tunnel: [w439 w443] -> w433
                frame False {
                  n126 = Build Array(w440) -> (w439:T4[])
                }
                frame True {
                  n127 = Build Array(T4 {"AlliGator Q Event"=enum."Phasor Graph:Save Phasor Graph Image", "Data"=variant} ("element"), w442) -> (w443:T4[])
                }
              }
              n128 = call "Hide Animated Busy Icon with Message.vi"("Already active? (F)"=w409, "Error In"=w422, "Target VI reference"=w410) -> ("Error Out"=w411:errorcluster)  [unwired: 8 in]
              n129 = call-poly "AlliGator Add Action(s) to Stack.vi"("Elements Order in Action Stack (Default: 2 BEFORE 1)"=Alligator_Elements_Order_in_Action_Stack."Enqueue 2 BEFORE 1", "Error In"=w411, "Alligator Queue Element 2"=w433, "Alligator Queue Element 1"=w438) -> ("Error Out"=w424:errorcluster, "Alligator Queue Element 1 (+ 2)"=w437:T4[])  [unwired: 6 in]
            }
          }
        }
      }
    }
    frame "Phasor Graph:Load Phasor Plot(s)" {
      # "#todo: handle Phasor SDV plots"
      # "\"Load Phasor Plot(s)\""
      n130 = Unbundle By Name(w451) -> ("Registered Events Ctrl Refnums.Phasor Graph"=w456:refnum<vi>)
      n131 = call-poly "Variant to Data.vi"("Variant"=w453) -> ("Value"=w452:path[])  [unwired: 8 in]
      n132 = call "Show Animated Busy Icon with Message.vi"("Already active? (F)"=w445, "Message"=w444, "Target VI Refnum"=w450) -> ("Error Out"=w455:errorcluster)  [unwired: 8 in]
      n133 = call "AlliGator Load Phasor Plot(s).vi"("Phasor Graph refnum"=w456, "error in (no error)"=w455, "File paths"=w452, "AlliGator IV DVR"=w448) -> ("error out"=w454:errorcluster, "Message"=w446:string, "AlliGator IV DVR"=w449:refnum<data-value>)  [unwired: 5 in]
      n134 = call "Hide Animated Busy Icon with Message.vi"("Already active? (F)"=w445, "Error In"=w454, "Target VI reference"=w450) -> ("Error Out"=w447:errorcluster)  [unwired: 8 in]
    }
    frame "Phasor Graph:Parameter 2 vs Parameter 1 Scatter Plot" {
      # "\"Phasor Graph:Parameter 2 vs Parameter 1 Scatter Plot\""
      n135 = Unbundle By Name(w470) -> ("Registered Events Ctrl Refnums.Lifetime Graph"=w458:refnum<vi>)
      n136 = Bundle("Selected Plot Info"=T14 {"Multiplot XY Graph"=refnum, "Mouse Coordinates"={"Horizontal"=0, "Vertical"=0}, "Plot Index"=-1}, "Scatter Plot Parameters"=T27 {"Parameter 2"=enum."Phasor g", "Parameter 1"=enum."Phasor g"}) -> (w464:T69)  [unwired: 1 in]
      n137 = Variant To Data(error in=w462, type=w464, Variant=w473) -> (data=w461:T69, error out=w469:errorcluster)
      n138 = call "AlliGator Compute P2 vs P1 Plots.vi"("Lifetime Graph in"=w458, "error in (no error)"=w469, "Phasor Frequency"=w459, "User Selection"=w461, "AlliGator IV DVR in"=w460) -> ("error out"=w466:errorcluster, "Message"=w467:string, "AlliGator IV DVR out"=w468:refnum<data-value>)  [unwired: 4 in]
    }
    frame "Phasor Graph:Phase Lifetime Trajectory" {
      # "Phase Lifetime Trajectory (deprecated)"
    }
    frame "Phasor Graph:Phase Lifetime vs Intensity Scatter Plot (deprecated)" {
      # "Phase Lifetime vs Intensity Scatter Plot (deprecated)"
    }
    frame "Phasor Graph:Phasor Multiplication" {
      # "\"Phasor Graph:Phasor Algebra\""
      n139 = Unbundle By Name(w491) -> ("Registered Events Ctrl Refnums.Phasor Graph"=w483:refnum<vi>)
      n140 = call "AlliGator Phasor Plot Multiplication Window.vi"("Phasor Graph"=w483) -> ("Error Out"=w489:errorcluster, "Cancelled"=w484:bool, "Phasor Plot Destination Output"=w482:T70, "Phasor Plot Algebra Output"=w490:T71)  [unwired: 7 in]
      n141 = case shown="False" w484 {
        tunnel: w490 -> [w495 _]
        tunnel: w489 -> [w501 w502]
        tunnel: [w500 w502] -> w488
        tunnel: [w499 w503] -> w487
        tunnel: w486 -> [w498 w503]
        tunnel: [w497 _] -> w485
        tunnel: w483 -> [w496 _]
        tunnel: w482 -> [w494 _]
        frame False {
          n142 = call "AlliGator Phasor Algebra Calculator.vi"("XYGraph in"=w496, "error in (no error)"=w501, "Phasor Plot Destination"=w494, "Phasor Plot Algebra Output"=w495, "Data Value Reference in"=w498) -> ("error out"=w500:errorcluster, "Message"=w497:string, "Data Value Reference out"=w499:refnum<data-value>)  [unwired: 4 in]
        }
        frame True {
        }
      }
    }
    frame "Phasor Graph:Python Function Phasor Graph Event" {
      # "\"Phasor Graph:Python Function Phasor Graph Event\""
      n143 = One Button Dialog(message="Not yet supported....") -> ()  [unwired: 1 in, 1 out]
      n144 = call "Play Error Sound.vi"() -> ()  [unwired: 27 in, 1 out]
    }
    frame "Phasor Graph:Remove Phasor Plot" {
      # "\"Phasor Graph:Remove Phasor Plot\""
      n145 = Variant To Data(Variant=w519) -> (data=w514:T14, error out=w513:errorcluster)  [unwired: 2 in]
      n146 = Unbundle By Name(w510) -> ("Phasor Graph Ctrl Refnums.Phasor Reference 1 Control"=w509:refnum<vi>)
      n147 = call "AlliGator Remove Phasor Plot.vi"("error in (no error)"=w513, "Phasor Reference 1 Refnum"=w509, "Selected Plot Info"=w514, "AlliGator IV DVR in"=w515) -> ("error out"=w512:errorcluster, "Message"=w511:string, "AlliGator IV DVR out"=w516:refnum<data-value>)  [unwired: 5 in]
    }
    frame "Phasor Graph:Remove Selected Phasor Plots" {
      # "\"Phasor Graph:Remove Selected Phasor Plots\""
      n148 = Variant To Data(Variant=w530) -> (data=w525:T14, error out=w524:errorcluster)  [unwired: 2 in]
      n149 = Unbundle By Name(w521) -> ("Phasor Graph Ctrl Refnums.Phasor Reference 1 Control"=w520:refnum<vi>)
      n150 = call "AlliGator Remove Selected Phasor Plots.vi"("error in (no error)"=w524, "Phasor Reference 1 Refnum"=w520, "Selected Plot Info"=w525, "AlliGator IV DVR in"=w526) -> ("error out"=w523:errorcluster, "Message"=w522:string, "AlliGator IV DVR out"=w527:refnum<data-value>)  [unwired: 5 in]
    }
    frame "Phasor Graph:Remove Single Phasor from Plot" {
      w531 = i32[] [0]  # Excludes UC
      # "Remove Single Phasor from Plot"
      n151 = Variant To Data(type=w533, Variant=w545) -> (data=w543:T17)  [unwired: 1 in, 1 out]
      n152 = Unbundle By Name(w543) -> ("Multiplot XY Graph"=w541:T15, "Mouse Coordinates"=w542:T16)
      n153 = call "XY Graph Remove Data Point.vi"("Excluded Plots"=w531, "Coords"=w542, "XYGraph in"=w541) -> ("Error Out"=w536:errorcluster, "Point  Index"=w538:i32, "Plot Number"=w539:i32, "Message"=w532:string, "Removed?"=w540:bool)  [unwired: 3 in, 1 out]
      n154 = case shown="True" w540 {
        tunnel: w539 -> [_ w550]
        tunnel: w538 -> [_ w549]
        tunnel: w534 -> [w546 w548]
        tunnel: [w546 w547] -> w535
        frame False {
        }
        frame True {
          n155 = in-place {
            in-place-border: w550 -> [w554]
            in-place-border: w549 -> [w553]
            n156 = in-place-dvr #5(w548) -> (w552:T33)  [unwired: 1 out]
            n157 = in-place {
              in-place-border: w554 -> [w558]
              in-place-border: w553 -> [w556]
              n158 = in-place-cluster #6(w552) -> ("[Phasor Graph:Raw Phasor Plots]"=w555:T51[])
              n159 = Decrement(x=w558) -> (x-1=w557:i32)
              n160 = call "AlliGator Manage Phasor Plots Array.vi"("[Raw Phasor Plot] in"=w555, "Plot Index (-1: Last)"=w557, "Phasor Index(-1: Last)"=w556, "[Raw Phasor Plot] Action"=AlliGator_Raw_Phasor_Plot_Array_Action."Remove Phasor in Plot") -> ("[Raw Phasor Plot] out"=w560:T51[])  [unwired: 15 in]
              n161 = in-place-cluster #6("[Phasor Graph:Raw Phasor Plots]"=w560) -> (w551:T33)
            }
            n162 = in-place-dvr #5(w551) -> (w547:refnum<data-value>)  [unwired: 1 out]
          }
        }
      }
    }
    frame "Phasor Graph:Save All Phasor Plots" {
      # "\"Save All Phasor Plots\""
      n163 = call-poly "Variant to Data.vi"("Variant"=w575) -> ("Value"=w574:bool)  [unwired: 8 in]
      n164 = Unbundle By Name(w569) -> ("Registered Events Ctrl Refnums.Phasor Graph"=w570:refnum<vi>)
      n165 = call "AlliGator IV [Raw Phasor Plot].vi"("Get (F)/ Set (T)"=FALSE, "AlliGator IV DVR in"=w568) -> ("error out"=w565:errorcluster, "[Raw Phasor Plots]"=w566:T51[], "AlliGator IV DVR out"=w567:refnum<data-value>)  [unwired: 7 in]
      n166 = Not(x=w574) -> (.not. x?=w573:bool)
      n167 = for {
        tunnel: w566 -> [w586] mode=indexing
        tunnel: w570 -> [w585]
        tunnel: w573 -> [w582]
        tunnel: [w580] -> w572 mode=indexing
        tunnel: w565 -> [w579]
        tunnel: [w578] -> w563 mode=indexing
        i -> [w584]
        w581 = TRUE  # Save as...
        n168 = Increment(x=w584) -> (x+1=w583:i32)
        n169 = call "AlliGator Save Raw Phasor v2.vi"("Save only if selected"=w582, "Save as..."=w581, "error in (no error)"=w579, "Raw Phasor Plot"=w586, "Selected Plot"=w583, "Phasor Graph"=w585) -> ("Error Out"=w580:errorcluster, "Message"=w578:string)  [unwired: 4 in]
      }
      n170 = Merge Errors(w572) -> (w571:errorcluster)
      n171 = call "Concatenate String Array.vi"("Separator (TAB)"="\r\n", "String Array"=w563) -> ("Formatted String"=w561:string)  [unwired: 9 in]
    }
    frame "Phasor Graph:Save Phasor Graph Image" {
      # "\"   Image\""
      n172 = call "AlliGator IV Dataset Path.vi"("Get (F)/ Set (T)"=FALSE, "error in (no error)"=w589, "AlliGator IV DVR in"=w600) -> ("error out"=w587:errorcluster, "[Time-Series Path]"=w597:path[], "Single Data Point Path"=w598:path, "AlliGator IV DVR out"=w599:refnum<data-value>, "Current Dataset"=w596:i32)  [unwired: 4 in]
      n173 = call "AlliGator Get Image File Format.vi"("Error In"=w589) -> ("error out"=w592:errorcluster, "File Extension (.xxx)"=w603:string, "Image File Format"=w602:T74)  [unwired: 7 in, 1 out]
      n174 = Unbundle By Name(w601) -> ("Registered Events Ctrl Refnums.Phasor Graph"=w604:refnum<vi>)
      n175 = Merge Errors(w587, w592) -> (w588:errorcluster)
      n176 = call "AlliGator Get Image Destination File Path.vi"("Image File Extension"=w603, "Image Name Prefix"="Phasor Graph " ("string"), "Error In"=w588, "Current Data Set"=w596, "Time-Series Paths"=w597, "Single Data Point Path"=w598) -> ("Error Out"=w591:errorcluster, "Image File Path"=w607:path)  [unwired: 4 in]
      n177 = call "XY Graph Save Graph Image.vi"("Error In"=w591, "Saved Image File Format"=w602, "Image File Path in"=w607, "XYGraph in"=w604) -> ("Error Out"=w593:errorcluster, "Image File Path out"=w606:path)  [unwired: 6 in]
      n178 = Path To String(path=w606) -> (string=w594:string)
    }
    frame "Phasor Graph:Save Single Phasor Plot" {
      # "\"Save Phasor Plot\""
      n179 = Variant To Data(type=T26 {"Mouse Click Event Data"={"Multiplot XY Graph"=refnum, "Mouse Coordinates"={"Horizontal"=0, "Vertical"=0}}, "Save as..."=FALSE} ("output cluster"), Variant=w627) -> (data=w626:T26, error out=w611:errorcluster)  [unwired: 1 in]
      n180 = Unbundle(w626) -> ("Mouse Click Event Data"=w625:T17, "Save as..."=w619:bool)
      n181 = call "AlliGator IV [Raw Phasor Plot].vi"("Get (F)/ Set (T)"=FALSE, "error in (no error)"=w611, "AlliGator IV DVR in"=w614) -> ("error out"=w610:errorcluster, "[Raw Phasor Plots]"=w613:T51[], "AlliGator IV DVR out"=w615:refnum<data-value>)  [unwired: 6 in]
      n182 = Unbundle(w625) -> ("Multiplot XY Graph"=w621:T15, "Mouse Coordinates"=w620:T16)
      n183 = call-poly "Get Plot at Mouse Click.vi"("error in (no error)"=w610, "Mouse Click Coordinates"=w620, "XYGraph Ref"=w621) -> ("error out"=w624:errorcluster, "Plot at Coordinates"=w617:i32, "XYGraph Ref"=w623:T15)  [unwired: 2 in, 4 out]
      n184 = case shown="-1, 1, Default" w617 {
        selector: w617 -> [_ w634]
        tunnel: w624 -> [w629 w642]
        tunnel: w623 -> [_ w643]
        tunnel: w619 -> [_ w641]
        tunnel: w613 -> [_ w633]
        tunnel: [w629 w639] -> w616
        tunnel: [_ w630] -> w609
        frame 0 {
          # "UC"
        }
        frame -1, 1, Default {
          # "UC is not part of Z plot array"
          n185 = Array Size(array=w633) -> (size(s)=w632:i32)
          n186 = Less Than 0?(x=w634) -> (x < 0?=w635:bool)
          n187 = Decrement(x=w634) -> (x-1=w636:i32)
          n188 = Select(t=w634, s=w635, f=w636) -> (s? t:f=w637:i32)
          n189 = Select(t=w632, s=w635, f=w634) -> (s? t:f=w631:i32)
          n190 = call "(Signed) Index 1D Array.vim"("Signed Index"=w637, "Array"=w633) -> ("Array Element"=w638:T51)  [unwired: 9 in]
          n191 = call "AlliGator IV Script Destination File Path.vi"() -> ("Destination File Path"=w640:path)
          n192 = call "AlliGator Save Raw Phasor v2.vi"("Save as..."=w641, "Phasor Plot Path (empty)"=w640, "error in (no error)"=w642, "Raw Phasor Plot"=w638, "Selected Plot"=w631, "Phasor Graph"=w643) -> ("Error Out"=w639:errorcluster, "Message"=w630:string)  [unwired: 4 in]
        }
      }
    }
    frame "Phasor Graph:Set Cursor n Location" {
      # "Set Cursor n Location"
      n193 = Variant To Data(type=T30 {"Current Phasor (g, s)"={"g"=0.0, "s"=0.0}, "Cursor Id"=0} ("output cluster"), Variant=w657) -> (data=w655:T30, error out=w653:errorcluster)  [unwired: 1 in]
      n194 = Unbundle By Name(w655) -> ("Cursor Id"=w650:u32, "Current Phasor (g, s)"=w654:T29)
      n195 = Unbundle By Name(w646) -> ("Registered Events Ctrl Refnums.Phasor Graph"=w647:refnum<vi>)
      n196 = Format Into String(format string=" (n = %d)", w650) -> (resulting string=w644:string)  [unwired: 2 in, 1 out]
      n197 = Decrement(x=w650) -> (x-1=w652:u32)
      n198 = property class="XYGraph (strict)"(reference=w647, error in=w653, "Active Cursor"=w652, "Cursor.Cursor Position"=w654) -> (error out=w648:errorcluster)  [unwired: 1 out]
    }
    frame "Phasor Graph:Set Reference n to Current Phase Lifetime Value" {
      # "\"Phasor Graph:Set Reference n to Current Phase Lifetime Value\""
      n199 = Unbundle By Name(w663) -> ("Phasor Graph Ctrl Refnums.Phase Lifetime"=w662:refnum<vi>)
      n200 = call-poly "Variant to Data.vi"("Variant"=w672) -> ("Value"=w665:i32)  [unwired: 8 in]
      n201 = property class="DigNum (strict)"(reference=w662) -> (error out=w660:errorcluster, "Value"=w661:dbl[unit])  [unwired: 1 in, 1 out]
      n202 = Format Into String(format string=" (n = %d)", w665) -> (resulting string=w659:string)  [unwired: 2 in, 1 out]
      n203 = case shown="No Error" w660 {
        tunnel: w671 -> [w691 w692]
        tunnel: [w690 w692] -> w670
        tunnel: w661 -> [w686 _]
        tunnel: w667 -> [w685 _]
        tunnel: [w684 _] -> w666
        tunnel: w665 -> [w675 _]
        frame No Error {
          n204 = call "Phasor Convert (tau, f) to (g, s) & (m, phi).vi"("Phasor Frequency"=w685, "Phase Lifetime"=w686) -> ("Error Out"=w684:errorcluster, "Phasor (g, s)"=w683:T29)  [unwired: 7 in, 1 out]
          n205 = Bundle("Phasor (g, s)"=w683, "Value"=w675) -> (w679:cluster{"Phasor (g, s)":T29, "Value":i32})  [unwired: 1 in]
          n206 = Build Array(w683) -> (w673:T29[])
          n207 = Bundle By Name(cluster=T31 {"Data Type"="Phasor Value", "Data"=variant} ("Phasor Reference Data"), "Data"=w679) -> (w677:T31)
          n208 = Bundle By Name(cluster=T4 {"AlliGator Q Event"=enum."Phasor Graph:Update Last Phasor Value", "Data"=variant} ("Alligator Atomic Action"), "Data"=w673) -> (w687:T4)
          n209 = Bundle By Name(cluster=T4 {"AlliGator Q Event"=enum."Phasor Ratio:Send Reference n to Notebook", "Data"=variant} ("Alligator Atomic Action"), "Data"=w675) -> (w674:T4)
          n210 = Bundle By Name(cluster=T4 {"AlliGator Q Event"=enum."Phasor Ratio:Use as Reference n", "Data"=variant} ("Alligator Atomic Action"), "Data"=w677) -> (w680:T4)
          n211 = Build Array(w687, w680, w674) -> (w681:T4[])
          n212 = call-poly "AlliGator Add Action(s) to Stack.vi"("Elements Order in Action Stack (Default: 2 BEFORE 1)"=Alligator_Elements_Order_in_Action_Stack."Enqueue 2 BEFORE 1", "Alligator Queue Element 2"=w681, "Alligator Queue Element 1"=w691) -> ("Alligator Queue Element 1 (+ 2)"=w690:T4[])  [unwired: 7 in, 1 out]
        }
        frame Error {
        }
      }
    }
    frame "Phasor Graph:Set Reference n to Lifetime Value" {
      # "Set Reference n to Lifetime Value"
      n213 = call-poly "Variant to Data.vi"("Variant"=w704) -> ("Value"=w695:i32)  [unwired: 8 in]
      n214 = Format Into String(format string=" (n = %d)", w695) -> (resulting string=w693:string)  [unwired: 2 in, 1 out]
      n215 = call "AlliGator Enter Reference Lifetime Dialog.vi"() -> ("Cancelled?"=w699:bool, "Reference Lifetime"=w698:dbl[unit])  [unwired: 9 in, 1 out]
      n216 = case shown="False" w699 {
        tunnel: w703 -> [w723 w724]
        tunnel: [w722 w724] -> w702
        tunnel: w698 -> [w718 _]
        tunnel: w697 -> [w717 _]
        tunnel: [w716 _] -> w696
        tunnel: w695 -> [w707 _]
        frame False {
          n217 = call "Phasor Convert (tau, f) to (g, s) & (m, phi).vi"("Phasor Frequency"=w717, "Phase Lifetime"=w718) -> ("Error Out"=w716:errorcluster, "Phasor (g, s)"=w715:T29)  [unwired: 7 in, 1 out]
          n218 = Bundle("Phasor (g, s)"=w715, "Value"=w707) -> (w711:cluster{"Phasor (g, s)":T29, "Value":i32})  [unwired: 1 in]
          n219 = Build Array(w715) -> (w705:T29[])
          n220 = Bundle By Name(cluster=T31 {"Data Type"="Phasor Value", "Data"=variant} ("Phasor Reference Data"), "Data"=w711) -> (w709:T31)
          n221 = Bundle By Name(cluster=T4 {"AlliGator Q Event"=enum."Phasor Graph:Update Last Phasor Value", "Data"=variant} ("Alligator Atomic Action"), "Data"=w705) -> (w719:T4)
          n222 = Bundle By Name(cluster=T4 {"AlliGator Q Event"=enum."Phasor Ratio:Send Reference n to Notebook", "Data"=variant} ("Alligator Atomic Action"), "Data"=w707) -> (w706:T4)
          n223 = Bundle By Name(cluster=T4 {"AlliGator Q Event"=enum."Phasor Ratio:Use as Reference n", "Data"=variant} ("Alligator Atomic Action"), "Data"=w709) -> (w712:T4)
          n224 = Build Array(w719, w712, w706) -> (w713:T4[])
          n225 = call-poly "AlliGator Add Action(s) to Stack.vi"("Elements Order in Action Stack (Default: 2 BEFORE 1)"=Alligator_Elements_Order_in_Action_Stack."Enqueue 2 BEFORE 1", "Alligator Queue Element 2"=w713, "Alligator Queue Element 1"=w723) -> ("Alligator Queue Element 1 (+ 2)"=w722:T4[])  [unwired: 7 in, 1 out]
        }
        frame True {
        }
      }
    }
    frame "Phasor Graph:Show Single Phasor" {
      # "\"Show Single Phasor\""
      n226 = Unbundle By Name(w731) -> ("Registered Events Ctrl Refnums.Phasor Graph"=w732:refnum<vi>)
      n227 = call "AlliGator IV Phasor Plot.vi"("Get (F)/ Set (T)"=FALSE, "AlliGator IV DVR in"=w730) -> ("Phasor Plot"=w728:cluster{"g Array":dbl[], "s Array":dbl[]}, "AlliGator IV DVR out"=w729:refnum<data-value>)  [unwired: 7 in, 1 out]
      n228 = call-poly "Variant to Data.vi"("Variant"=w739) -> ("Value"=w738:i32)  [unwired: 8 in]
      n229 = case shown="0, Default" w738 {
        selector: w738 -> [_ w773]
        tunnel: [w741 w770] -> w737
        tunnel: [w742 w760] -> w735
        tunnel: w728 -> [w741 w764]
        tunnel: w726 -> [w740 w763]
        tunnel: [w740 w762] -> w725
        frame ..-1 {
          # "Show the whole phasor plot"
          n230 = xnode "Error Ring"() -> ("error out"=w745:errorcluster)
          n231 = Unbundle By Name(w741) -> ("g Array"=w743:dbl[])
          n232 = xnode "Error Ring"() -> ("error out"=w744:errorcluster)
          n233 = Empty Array?(array=w743) -> (empty?=w746:bool)
          n234 = Select(t=w745, s=w746, f=w744) -> (s? t:f=w742:errorcluster)
        }
        frame 0, Default {
          n235 = Unbundle By Name(w764) -> ("g Array"=w768:dbl[], "s Array"=w774:dbl[])
          n236 = Decrement(x=w773) -> (x-1=w769:i32)
          n237 = xnode "Error Ring"() -> ("error out"=w766:errorcluster)
          n238 = Index Array(array=w768, index=w769) -> (element=w756:dbl)
          n239 = Index Array(array=w774, index=w769) -> (element=w755:dbl)
          n240 = Bundle By Name(cluster=T29 {"g"=0.0, "s"=0.0} ("Phasor"), "g"=w756, "s"=w755) -> (w753:T29)
          n241 = xnode "Error Ring"() -> ("error out"=w765:errorcluster)
          n242 = Build Array(w753) -> (w752:T29[])
          n243 = Build Array(w756) -> (w772:dbl[])
          n244 = Empty Array?(array=w768) -> (empty?=w767:bool)
          n245 = Build Array(w755) -> (w771:dbl[])
          n246 = Bundle By Name(cluster=T4 {"AlliGator Q Event"=enum."Phasor Graph:Update Last Phasor Value", "Data"=variant} ("Alligator Atomic Action"), "Data"=w752) -> (w757:T4)
          n247 = Select(t=w766, s=w767, f=w765) -> (s? t:f=w761:errorcluster)
          n248 = Bundle(w772, w771) -> (w770:cluster{dbl[], dbl[]})  [unwired: 1 in]
          n249 = call-poly "AlliGator Add Action(s) to Stack.vi"("Elements Order in Action Stack (Default: 2 BEFORE 1)"=Alligator_Elements_Order_in_Action_Stack."Enqueue 2 BEFORE 1", "Error In"=w761, "Alligator Atomic Action"=w757, "Alligator Queue Element 1"=w763) -> ("Error Out"=w760:errorcluster, "Alligator Queue Element 1 (+ 2)"=w762:T4[])  [unwired: 6 in]
        }
      }
      n250 = call "XY Graph Insert Plot.vi"("Error In"=w735, "Plot Index (Default Inf: Append to End)"=-1, "New Plot"=w737, "Multiplot XY Graph Refnum in"=w732) -> ("Error Out"=w733:errorcluster)  [unwired: 5 in, 2 out]
    }
    frame "Phasor Graph:Update Last Phasor Value" {
      w780 = TRUE ("Get (F)/ Set (T)")
      # "\"Update Last Phasor Value\""
      n251 = Unbundle By Name(w792) -> ("Phasor Graph Ctrl Refnums"=w791:T9)
      n252 = Variant To Data(type=T29[] [] ("Phasor"), Variant=w797) -> (data=w789:T29[], error out=w793:errorcluster)  [unwired: 1 in]
      n253 = Index Array(array=w789) -> (element #1=w787:T29, element #2=w781:T29)  [unwired: 2 in]
      n254 = call "AlliGator Update Phasor Graph Information at Cursor.vi"("Valid?"=TRUE, "Error In"=w793, "Phasor SDV"=w781, "Phasor"=w787, "Current Phasor Information Indicators"=w791) -> ("Error Out"=w788:errorcluster)  [unwired: 5 in, 1 out]
      n255 = call "AlliGator IV Last Calibrated Phasor.vi"("Get (F)/ Set (T)"=w780, "error in (no error)"=w788, "Last Calibrated Phasor"=w787, "AlliGator IV DVR in"=w790) -> ("error out"=w783:errorcluster, "AlliGator IV DVR out"=w785:refnum<data-value>)  [unwired: 5 in, 1 out]
      n256 = call "AlliGator IV Last Calibrated Phasor SDV.vi"("Get (F)/ Set (T)"=w780, "error in (no error)"=w783, "Last Calibrated Phasor SDV"=w781, "AlliGator IV DVR in"=w785) -> ("error out"=w782:errorcluster, "AlliGator IV DVR out"=w784:refnum<data-value>)  [unwired: 5 in, 1 out]
    }
    frame "Phasor Graph:Update Phasor (m, phi)" {
      # "\"Updated Phasor (m, phi)\""
      n257 = Unbundle By Name(w806) -> ("Phasor Graph Ctrl Refnums"=w805:T9)
      n258 = Variant To Data(type=T32 {"m"=0.0, "phi"=0.0} ("Phasor"), Variant=w812) -> (data=w809:T32, error out=w807:errorcluster)  [unwired: 1 in]
      n259 = call "Phasor Convert (m, phi) to (g,s).vi"("Phasor (m, phi)"=w809) -> ("Phasor (g, s)"=w802:T29)  [unwired: 8 in]
      n260 = call "AlliGator Update Phasor Graph Information at Cursor.vi"("Valid?"=TRUE, "Error In"=w807, "Phasor"=w802, "Current Phasor Information Indicators"=w805) -> ("Error Out"=w801:errorcluster)  [unwired: 6 in, 1 out]
      n261 = call "AlliGator IV Last Calibrated Phasor.vi"("Get (F)/ Set (T)"=TRUE, "error in (no error)"=w801, "Last Calibrated Phasor"=w802, "AlliGator IV DVR in"=w803) -> ("error out"=w800:errorcluster, "AlliGator IV DVR out"=w804:refnum<data-value>)  [unwired: 5 in, 1 out]
    }
    frame "Phasor Graph:Update SEPL Plot" {
      w816 = i32[] [5001, 5025, 5026]  # Not a Valid Plot, Incompatible References
      # "\"Update SEPL Plot\""
      n262 = call "Show Animated Busy Icon with Message.vi"("Already active? (F)"=w815, "Message"=w813, "Error In"=w814, "Target VI Refnum"=w818) -> ("Error Out"=w830:errorcluster)  [unwired: 7 in]
      n263 = Unbundle By Name(w820) -> ("Other AlliGator Ctrl Refnums.State Indicators"=w819:refnum<vi>, "Registered Events Ctrl Refnums.Phasor Graph"=w827:refnum<vi>)
      n264 = call "AlliGator Compute SEPL Plot.vi"("Error In"=w830) -> ("error out"=w832:errorcluster, "SEPL Plot"=w834:cluster{"X Array":dbl[], "Y Array":dbl[]}, "Plot Name"=w831:string)  [unwired: 7 in, 1 out]
      n265 = call "XY Graph Update Plot.vi"("New Plot Name (Default: unchanged)"=w831, "Error In"=w832, "Plot"=w834, "Plot Idx"=0 ("Plot Index (Default Inf: Append to End)"), "XY Graph refnum"=w827) -> ("Error Out"=w825:errorcluster)  [unwired: 6 in]
      n266 = call "AlliGator Get Updated Phasor Ratio References.vi"("error in (no error)"=w825) -> ("error out"=w822:errorcluster, "Phasor Ratio Reference 2"=w823:T29, "Phasor Ratio Reference 1"=w824:T29)  [unwired: 8 in]
      n267 = call "AlliGator Define Phasor References.vi"("Phasor Graph"=w827, "State Indicators Refnum"=w819, "Phasor 1"=w824, "Phasor 2"=w823, "Phasor Frequency"=w826, "Error In"=w822) -> ("Error Out"=w828:errorcluster)  [unwired: 5 in, 4 out]
      n268 = call "Hide Animated Busy Icon with Message.vi"("Already active? (F)"=w815, "Error In"=w828, "Target VI reference"=w818) -> ("Error Out"=w829:errorcluster)  [unwired: 8 in]
      n269 = call "Filter Errors.vi"("Filtered Errors"=w816, "error in (no error)"=w829) -> ("error out"=w821:errorcluster)  [unwired: 7 in]
    }
    frame "Phasor Graph:Use Cursor n Location" {
      # "Cursor #"
      # "\"Use Cursor n Location\""
      n270 = call-poly "Variant to Data.vi"("Variant"=w852) -> ("Value"=w844:u32)  [unwired: 8 in]
      n271 = Format Into String(format string=" (n = %d)", w844) -> (resulting string=w836:string)  [unwired: 2 in, 1 out]
      n272 = Unbundle By Name(w839) -> ("Registered Events Ctrl Refnums.Phasor Graph"=w840:refnum<vi>)
      n273 = Decrement(x=w844) -> (x-1=w845:u32)
      n274 = property class="XYGraph (strict)"(reference=w840, "Active Cursor"=w845) -> (error out=w841:errorcluster, "Cursor.Cursor Position"=w846:T75)  [unwired: 1 in, 1 out]
      n275 = Build Array(w846) -> (w837:T75[])
      n276 = Bundle By Name(cluster=T4 {"AlliGator Q Event"=enum."Phasor Graph:Update Last Phasor Value", "Data"=variant} ("Alligator Atomic Action"), "Data"=w837) -> (w847:T4)
      n277 = call-poly "AlliGator Add Action(s) to Stack.vi"("Elements Order in Action Stack (Default: 2 BEFORE 1)"=Alligator_Elements_Order_in_Action_Stack."Enqueue 2 BEFORE 1", "Alligator Atomic Action"=w847, "Alligator Queue Element 1"=w851) -> ("Alligator Queue Element 1 (+ 2)"=w850:T4[])  [unwired: 7 in, 1 out]
    }
    frame "Phasor Graph:Use Selected Plots Fitted Line/UC Intersections" {
      # "\"Phasor Graph: Use Selected Plots Fitted Line/UC Intersections\""
      n278 = Variant To Data(type=T15 refnum ("Multiplot XY Graph"), Variant=w889) -> (data=w876:T15, error out=w875:errorcluster)  [unwired: 1 in]
      n279 = Unbundle By Name(w866) -> ("Other AlliGator Ctrl Refnums.State Indicators"=w878:refnum<vi>, "Phasor Graph Ctrl Refnums.Phase Lifetime 1"=w865:refnum<vi>, "Phasor Graph Ctrl Refnums.Phase Lifetime 2"=w864:refnum<vi>, "Phasor Graph Ctrl Refnums.Show Line"=w863:refnum<vi>)
      n280 = call "Show Animated Busy Icon with Message.vi"("Already active? (F)"=w854, "Error In"=w875, "Target VI Refnum"=w856) -> ("Error Out"=w858:errorcluster)  [unwired: 8 in]
      n281 = call "XY Graph Get Selected Plot Names & Indices.vi"("error in (no error)"=w858, "XYGraph in"=w876) -> ("error out"=w874:errorcluster, "Selected Plots"=w869:i32[], "Selected Plot Names"=w873:string[])  [unwired: 5 in, 2 out]
      n282 = call-poly <userlib>:"Filter 1D Array__ogtk.vi"("items to filter"=0, "array"=w869) -> ("filtered array"=w868:i32[])  [unwired: 4 in, 1 out]
      n283 = call "Concatenate String Array.vi"("Separator (TAB)"=", ", "Suffix (\"\")"="):" ("Suffix (\"\")"), "String Array"=w873, "Prefix (\"\")"=" (" ("Prefix (\"\")")) -> ("Formatted String"=w853:string)  [unwired: 7 in]
      n284 = for {
        tunnel: [w895] -> w880 mode=concatenating
        tunnel: w876 -> [w893]
        tunnel: w874 -> [w892]
        tunnel: [w894] -> w879
        tunnel: w868 -> [w891] mode=indexing
        n285 = call "AlliGator Get Phasor Plot Data.vi"("error in (no error)"=w892, "Plot Idx (-1: last)"=w891, "Phasor Graph Refnum"=w893) -> ("error out"=w894:errorcluster, "Phasor Array"=w895:T29[])  [unwired: 5 in, 2 out]
      }
      n286 = call "Phasor Find Intersections of Fitted Line with Universal Circle.vi"("Error In"=w879, "Phasor Array"=w880) -> ("Error Out"=w882:errorcluster, "Intersection 2"=w883:T29, "Intersection 1"=w884:T29)  [unwired: 7 in]
      n287 = Unbundle By Name(w882) -> ("status"=w881:bool)
      n288 = call "AlliGator Define Phasor References.vi"("Phasor Graph"=w876, "State Indicators Refnum"=w878, "Phasor 1"=w884, "Phasor 2"=w883, "Phasor Frequency"=w859, "Error In"=w882) -> ("Reference Lifetime 1"=w888:dbl[unit], "Reference Lifetime 2"=w887:dbl[unit], "Phasor Reference 1"=w886:T29, "Phasor Reference 2"=w885:T29, "Error Out"=w862:errorcluster)  [unwired: 5 in]
      n289 = Not(x=w881) -> (.not. x?=w860:bool)
      n290 = call "Hide Animated Busy Icon with Message.vi"("Already active? (F)"=w854, "Error In"=w862, "Target VI reference"=w856) -> ("Error Out"=w857:errorcluster)  [unwired: 8 in]
      n291 = property class="Bool (strict)"(reference=w863, error in=w857, "Val(Sgnl)"=w860) -> (error out=w861:errorcluster)  [unwired: 1 out]
      n292 = case shown="No Error" w857 {
        tunnel: w888 -> [w898 _]
        tunnel: w887 -> [w897 _]
        tunnel: w886 -> [_ _]
        tunnel: w885 -> [_ _]
        tunnel: w865 -> [w900 _]
        tunnel: w864 -> [w899 _]
        frame No Error {
          w896 = TRUE ("Visible")
          n293 = property class="DigNum (strict)"(reference=w900, "Value"=w898, "Visible"=w896) -> ()  [unwired: 1 in, 2 out]
          n294 = property class="DigNum (strict)"(reference=w899, "Value"=w897, "Visible"=w896) -> ()  [unwired: 1 in, 2 out]
        }
        frame Error {
        }
      }
    }
    frame "Phasor Graph:Use Selected Plots Principal Axis/UC Intersections" {
      # "\"Phasor Graph: Use Selected Plots Principal Axis/UC Intersections\""
      n295 = call-poly "Variant to Data.vi"("Variant"=w921) -> ("Value"=w918:bool)  [unwired: 8 in]
      n296 = Unbundle By Name(w916) -> ("Registered Events Ctrl Refnums.Phasor Graph"=w909:refnum<vi>, "Phasor Graph Ctrl Refnums.Phase Lifetime 1"=w915:refnum<vi>, "Phasor Graph Ctrl Refnums.Phase Lifetime 2"=w914:refnum<vi>, "Other AlliGator Ctrl Refnums.State Indicators"=w908:refnum<vi>, "Phasor Graph Ctrl Refnums.Show Line"=w910:refnum<vi>)
      n297 = call "XY Graph Get Selected Plot Names & Indices.vi"("XYGraph in"=w909) -> ("error out"=w928:errorcluster, "Selected Plots"=w920:i32[], "Selected Plot Names"=w927:string[], "XYGraph out"=w919:T15)  [unwired: 6 in, 1 out]
      n298 = call-poly <userlib>:"Filter 1D Array__ogtk.vi"("items to filter"=0, "array"=w920) -> ("filtered array"=w923:i32[])  [unwired: 4 in, 1 out]
      n299 = call "Concatenate String Array.vi"("Separator (TAB)"=", ", "Suffix (\"\")"="):" ("Suffix (\"\")"), "String Array"=w927, "Prefix (\"\")"=" (" ("Prefix (\"\")")) -> ("Formatted String"=w917:string)  [unwired: 7 in]
      n300 = call "Show Animated Busy Icon with Message.vi"("Already active? (F)"=w901, "Error In"=w928, "Target VI Refnum"=w904) -> ("Error Out"=w906:errorcluster)  [unwired: 8 in]
      n301 = call "AlliGator Use Phasor Graph Selected Phasor Plots Principal Axis - UC Intersections as References.vi"("Selected Plot List"=w917, "error in (no error)"=w906, "Major Axis?"=w918, "Selected Plot Indices"=w923, "Phasor Graph refnum"=w919) -> ("error out"=w930:errorcluster, "Message"=w902:string, "Intersection 1"=w932:cluster{"x":dbl, "y":dbl}, "Intersection 2"=w931:cluster{"x":dbl, "y":dbl})  [unwired: 3 in]
      n302 = call "Hide Animated Busy Icon with Message.vi"("Already active? (F)"=w901, "Error In"=w930, "Target VI reference"=w904) -> ("Error Out"=w905:errorcluster)  [unwired: 8 in]
      n303 = Unbundle By Name(w905) -> ("status"=w929:bool)
      n304 = call "AlliGator Define Phasor References.vi"("Phasor Graph"=w909, "State Indicators Refnum"=w908, "Phasor 1"=w932, "Phasor 2"=w931, "Phasor Frequency"=w907, "Error In"=w905) -> ("Reference Lifetime 1"=w936:dbl[unit], "Reference Lifetime 2"=w935:dbl[unit], "Phasor Reference 1"=w934:T29, "Phasor Reference 2"=w933:T29, "Error Out"=w912:errorcluster)  [unwired: 5 in]
      n305 = Not(x=w929) -> (.not. x?=w913:bool)
      n306 = case shown="No Error" w912 {
        tunnel: w936 -> [w941 _]
        tunnel: w935 -> [w939 _]
        tunnel: w934 -> [_ _]
        tunnel: w933 -> [_ _]
        tunnel: w915 -> [w942 _]
        tunnel: w914 -> [w940 _]
        frame No Error {
          w938 = TRUE ("Visible")
          n307 = property class="DigNum (strict)"(reference=w942, "Value"=w941, "Visible"=w938) -> ()  [unwired: 1 in, 2 out]
          n308 = property class="DigNum (strict)"(reference=w940, "Value"=w939, "Visible"=w938) -> ()  [unwired: 1 in, 2 out]
        }
        frame Error {
        }
      }
      n309 = property class="Bool (strict)"(reference=w910, error in=w912, "Val(Sgnl)"=w913) -> (error out=w911:errorcluster)  [unwired: 1 out]
    }
    frame "Phasor Graph:Use UC/Cursor-Defined Line Intersections" {
      w945 = TRUE ("Visible")
      # "Use UC/Cursor-Defined Line Intersections"
      n310 = Unbundle By Name(w948) -> ("Phasor Graph Ctrl Refnums.Phase Lifetime 1"=w952:refnum<vi>, "Phasor Graph Ctrl Refnums.Phase Lifetime 2"=w951:refnum<vi>, "Other AlliGator Ctrl Refnums.State Indicators"=w953:refnum<vi>, "Registered Events Ctrl Refnums.Phasor Graph"=w954:refnum<vi>)  [unwired: 1 out]
      n311 = Unbundle By Name(w948) -> ("Phasor Graph Ctrl Refnums.Phasor Reference 1 Control"=w947:refnum<vi>)
      n312 = call "AlliGator Find Cursor Connecting Line Intersection(s) with Universal Circle.vi"("XY Graph Refnum"=w954) -> ("Error Out"=w958:errorcluster, "Intersection 2"=w959:cluster{"x":dbl, "y":dbl}, "Intersection 1"=w960:cluster{"x":dbl, "y":dbl})  [unwired: 8 in]
      n313 = call "AlliGator Define Phasor References.vi"("Phasor Graph"=w954, "State Indicators Refnum"=w953, "Phasor 1"=w960, "Phasor 2"=w959, "Phasor Frequency"=w956, "Error In"=w958) -> ("Reference Lifetime 1"=w950:dbl[unit], "Reference Lifetime 2"=w949:dbl[unit], "Error Out"=w943:errorcluster)  [unwired: 5 in, 2 out]
      n314 = call "Phasor Convert (tau, f) to (m, phi).vi"("Lifetime"=w950, "Phasor Frequency"=w956) -> ("Phasor (m, phi)"=w957:T32)  [unwired: 5 in]
      n315 = property class="DigNum (strict)"(reference=w952, "Value"=w950, "Visible"=w945) -> ()  [unwired: 1 in, 2 out]
      n316 = property class="DigNum (strict)"(reference=w951, "Value"=w949, "Visible"=w945) -> ()  [unwired: 1 in, 2 out]
      n317 = Unbundle By Name(w957) -> ("phi"=w946:dbl)
      n318 = property class="Scroll (strict)"(reference=w947, "Value"=w946) -> ()  [unwired: 1 in, 2 out]
    }
    frame "Phasor Graph:Whole Image Phasor Scatter Plot (Todo)" {
      # "\"Phasor Graph:Whole Image Phasor Scatter Plot (Todo)\""
      n319 = disable-structure shown="Enabled" {
        disable-tunnel: w966 -> [w973 w974]
        disable-tunnel: [w972 w974] -> w965
        disable-tunnel: [w967 _] -> w963
        frame Disabled {
          n320 = Bundle By Name(cluster=T4 {"AlliGator Q Event"=enum."Phasor Graph:Whole Image Phasor Scatter Plot (Todo)", "Data"=variant} ("element"), "Data"=-1) -> (w969:T4)
          n321 = call-poly "AlliGator Add Action(s) to Stack.vi"("Elements Order in Action Stack (Default: 2 BEFORE 1)"=Alligator_Elements_Order_in_Action_Stack."Enqueue 2 BEFORE 1", "Alligator Atomic Action"=w969, "Alligator Queue Element 1"=w973) -> ("Error Out"=w967:errorcluster, "Alligator Queue Element 1 (+ 2)"=w972:T4[])  [unwired: 7 in]
        }
        frame Enabled {
          # "#Todo\nwrite a script that:\n- temporarily save current ROI list (and selected ROI)\n- delete all ROIs\n- create all pixels ROIs\n- run the all ROIs Phasor Analysis script\n- delete all ROIs\n- restore intial ROIs\n- restore selected ROI"
        }
      }
    }
  }
  "Data Value Reference out" <- w19
  "error out" <- w8
  "Script out" <- w11
  "AlliGator Q Elements out" <- w10
  n322 = call "Message Style.vi"() -> ("Message Formatting"=w3:T2)
  n323 = call "AlliGator Package Notebook Messages.vi"("Message Formatting"=w3, "Message"=w2, "AlliGator Q Event in"="AlliGator Q Event in") -> ("[Notebook Message]"=→"[Notebook Message]":T1[])  [unwired: 8 in]
